vi "WS102x FPGA Multi DUT Reliability Ver1.1.vi"() -> ()   [LabVIEW 2017]
uses:
  Type Def/Test Sequences.ctl
  WS_VCAP Driver 039/Source/WSVCAP Shell/Type Defs/WSVCAP SHL FPGA Enum.ctl
  <vilib>/userdefined/High Color/nirio_resource_hc.ctl
  WS_VCAP Driver 039/Source/WSVCAP Shell/Type Defs/WSVCAP SHL I2C DUT Mask Mode Enum.ctl
  <vilib>/Utility/error.llb/whitespace.ctl
  <vilib>/Utility/file.llb/Read Delimited Spreadsheet (DBL).vi
panel:
  in  "Main":T1(tab)
  in  "Clock Rate Meas(Hz)":dbl=1000000.0 format="%.1p Hz"
  in  "CAPDAC Value":u8=128 format="0x%02x"
  in  "DUT Mask Mode (All)":T2=enum."All"
  in  "SN Brd B":string[](array[string])=["1", "2", "3", "4", "5", "6", "7", "8", "9", "10", "11", "12", "13", "14", "15", "16", "17", "18", "19", "20", "21", "22", "23", "24", "25", "26", "27", "28", "29", "30", "31", "32"]
  in  "SN Brd A":string[](array[string])=["1", "2", "3", "4", "5", "6", "7", "8", "9", "10", "11", "12", "13", "14", "15", "16", "17", "18", "19", "20", "21", "22", "23", "24", "25", "26", "27", "28", "29", "30", "31", "32"]
  in  "Info Brd B":T3={"Lot #"="1K3CB", "Wafer #"="19", "Board"="B", "Comment"="CYC 45C 44V", "File Name"="CYC_1K3CB_19WO_25C_44V_25DC_Brd2B_190124_1", "Data File Path Control"=path "C:/WS102x 32 DUT Data"}
  in  "Info Brd A":T3={"Lot #"="1K3CB", "Wafer #"="19", "Board"="A", "Comment"="CYC 45C 44V", "File Name"="CYC_1K3CB_19_WO_25C_44V_25DC_Brd2A_190124_1", "Data File Path Control"=path "C:/WS102x 32 DUT Data"}
  in  "Test Program":string="WS102x FPGA Multi DUT Reliability Ver1.1"
  in  "Calibration AD":bool
  in  "Initialize ADI":bool
  in  "Data Brd B?":bool=TRUE
  in  "Data Brd A?":bool=TRUE
  in  "Setup Test":T4(tab)
  in  "Manual Command":string
  in  "Verify Beams":bool
  in  "Manual Setting":i32(ring) items=["CP OFF", "CP ON", "OTP OFF", "CP 24V", "CP 26V", "CP 28V", "CP 30V", "CP 31V", "CP 32V", "CP 33V", "CP 34V", "CP 35V", "CP 36V", "CP 37V", "CP 38V", "CP 39V", "CP 40V", "CP 41V", "CP 42V", "CP 43V", "CP 44V", "CP 45V", "CP 46V", "CP 47V", "CP 48V", "CP 49V", "CP 50V", "CP 51V", "CP 52V", "CP 53V", "CP 54V", "CP 56V", "CP 58V", "CP 60V", "CP 62V"]
  in  "CP Measurement":i32(ring)=20 items=["CP OFF", "CP ON", "OTP OFF", "CP 24V", "CP 26V", "CP 28V", "CP 30V", "CP 31V", "CP 32V", "CP 33V", "CP 34V", "CP 35V", "CP 36V", "CP 37V", "CP 38V", "CP 39V", "CP 40V", "CP 41V", "CP 42V", "CP 43V", "CP 44V", "CP 45V", "CP 46V", "CP 47V", "CP 48V", "CP 49V", "CP 50V", "CP 51V", "CP 52V", "CP 53V", "CP 54V", "CP 56V", "CP 58V", "CP 60V", "CP 62V"]
  in  "Select CP VPI":i32(ring)=16 items=["CP OFF", "CP ON", "OTP OFF", "CP 24V", "CP 26V", "CP 28V", "CP 30V", "CP 31V", "CP 32V", "CP 33V", "CP 34V", "CP 35V", "CP 36V", "CP 37V", "CP 38V", "CP 39V", "CP 40V", "CP 41V", "CP 42V", "CP 43V", "CP 44V", "CP 45V", "CP 46V", "CP 47V", "CP 48V", "CP 49V", "CP 50V", "CP 51V", "CP 52V", "CP 53V", "CP 54V", "CP 56V", "CP 58V", "CP 60V", "CP 62V"]
  in  "Select CP Stress":i32(ring)=20 items=["CP OFF", "CP ON", "OTP OFF", "CP 24V", "CP 26V", "CP 28V", "CP 30V", "CP 31V", "CP 32V", "CP 33V", "CP 34V", "CP 35V", "CP 36V", "CP 37V", "CP 38V", "CP 39V", "CP 40V", "CP 41V", "CP 42V", "CP 43V", "CP 44V", "CP 45V", "CP 46V", "CP 47V", "CP 48V", "CP 49V", "CP 50V", "CP 51V", "CP 52V", "CP 53V", "CP 54V", "CP 56V", "CP 58V", "CP 60V", "CP 62V"]
  in  "VDD":dbl=3.3 format="%.2g"
  in  "CP Setting":bool
  in  "Cycle DC %":string="25"
  in  "Set Delay Speed":dbl[](array[numeric])=[1.7e-05, 4.9e-05] min=0.0 max=0.5 format="%#.0p s"
  in  "Cycling Bit":string[](array[string])=["0701027F7F", "0701020000"]
  out "Stress DC(%)":string
  in  "HD Beams":string="ALL Beams"
  in  "HD Cmd":string="0701027F7F"
  in  "Test Condition Setting":T5={"Freq (KHz)"="12", "ACV (V)"="0", "AC Freq (Hz)"="0", "Temp (C)"="25", "DCV (V)"=0.0, "CYC RP (x1000)"=10000, "HD RP (Min)"=60, "RPM Delay (s)"=60, "Select VCmin"=2} {"Select VCmin" items=["FBs", "TBs", "ALL"]}
  out "Test Run Selected":T6
  in  "Test Run Setting":T7={"OTP ?  "=FALSE, "STRESS ?  "=TRUE, "VPI ?  "=TRUE, "OPEN STATE VCMIN ?  "=TRUE, "CLOSE STATE VCMIN ?  "=TRUE, "RPM (Verify Socket) ?  "=FALSE, "HS CHK?"=TRUE}
  out "Data Board B":string[][](array[string])
  in  "Stop":bool
  out "Current Time":string
  out "Current Date":string
  in  "Start Date":string
  in  "Start Time":string
  in  "Select Measurement":i32(ring) items=["Temperature", "Humidity", "TH1", "TH2"]
  out "Temp (C)":string
  out "RH(%)":string
  out "Test Sequences":T8
  out "Error Out":errorcluster
  in  "Error In":errorcluster
  in  "Start":bool
  out "Data Board A":string[][](array[string])
  out "AD7747 Value Brd B":string[][](table)=[["Device", "Status", "Cap (pF)", "SN"], ["DUT 01", "", "", "01"], ["DUT 02", "", "", "02"], ["DUT 03", "", "", "03"], ["DUT 04", "", "", "04"], ["DUT 05", "", "", "05"], ["DUT 06", "", "", "06"], ["DUT 07", "", "", "07"], ["DUT 08", "", "", "08"], ["DUT 09", "", "", "09"], ["DUT 10", "", "", "10"], ["DUT 11", "", "", "11"], ["DUT 12", "", "", "12"], ["DUT 13", "", "", "13"], ["DUT 14", "", "", "14"], ["DUT 15", "", "", "15"], ["DUT 16", "", "", "16"], ["DUT 17", "", "", "17"], ["DUT 18", "", "", "18"], ["DUT 19", "", "", "19"], ["DUT 20", "", "", "20"], ["DUT 21", "", "", "21"], ["DUT 22", "", "", "22"], ["DUT 23", "", "", "23"], ["DUT 24", "", "", "24"], ["DUT 25", "", "", "25"], ["DUT 26", "", "", "26"], ["DUT 27", "", "", "27"], ["DUT 28", "", "", "28"], ["DUT 29", "", "", "29"], ["DUT 30", "", "", "30"], ["DUT 31", "", "", "31"], ["DUT 32", "", "", "32"]]
  out "AD7747 Value Brd A":string[][](table)=[["Device", "Status", "Cap (pF)", "SN"], ["DUT 01", "", "", "01"], ["DUT 02", "", "", "02"], ["DUT 03", "", "", "03"], ["DUT 04", "", "", "04"], ["DUT 05", "", "", "05"], ["DUT 06", "", "", "06"], ["DUT 07", "", "", "07"], ["DUT 08", "", "", "08"], ["DUT 09", "", "", "09"], ["DUT 10", "", "", "10"], ["DUT 11", "", "", "11"], ["DUT 12", "", "", "12"], ["DUT 13", "", "", "13"], ["DUT 14", "", "", "14"], ["DUT 15", "", "", "15"], ["DUT 16", "", "", "16"], ["DUT 17", "", "", "17"], ["DUT 18", "", "", "18"], ["DUT 19", "", "", "19"], ["DUT 20", "", "", "20"], ["DUT 21", "", "", "21"], ["DUT 22", "", "", "22"], ["DUT 23", "", "", "23"], ["DUT 24", "", "", "24"], ["DUT 25", "", "", "25"], ["DUT 26", "", "", "26"], ["DUT 27", "", "", "27"], ["DUT 28", "", "", "28"], ["DUT 29", "", "", "29"], ["DUT 30", "", "", "30"], ["DUT 31", "", "", "31"], ["DUT 32", "", "", "32"]]
  in  "Instruments":T10={"KE2400"="GPIB0::3::INSTR", "KE2000"="GPIB0::9::INSTR", "Agilent P/S"="GPIB0::5::INSTR", "Temperature Sensor"="", "FPGA"=enum."RIO0"}
  out "Activity Log":string
  out "FPGA Resource":T11
  out "Online":bool
  out "Simulate FPGA":bool
  in  "RFFE Slave Address":u8=7 caption="Slave Address" format="0x%02x"
  in  "Clock Rate Cycle(Hz)":dbl=5000000.0 format="%.1p Hz"
  out "Error Status":string
  out "IDD Measurement(uA)":string[](array[string])
  out "Cycle Count":u64=2 min=1 max=4 step=1
  out "Status":string
  out "Last Run Time":string
  out "Last Run Date":string
  out "T0_Brd B Delta C%":string[](array[string])
  out "T0_Brd A Delta C%":string[](array[string])
  in  "Abort Stress":bool
  out "TTF Completed":u64
  in  "Set TTF":u64=50000000000
  out "Brd B_VPI Cap (fF)":string[][](table)
  out "Brd B_Beam Cap (fF)":string[][](table)
  out "Brd A_VPI Cap (fF)":string[][](table)
  out "Brd A_Beam Cap (fF)":string[][](table)
  out "Verify CP Stress":string[](array[string])
  out "Brd B Pass/Fail?":bool[](array[boolean])
  out "Brd A Pass/Fail?":bool[](array[boolean])
  out "Verify DC Speed":dbl[](array[numeric]) format="%#.0p s"
  out "Verify Bits to Cycle":string[](array[string])
  out "Brd A Delta C%":string[](array[string])
  out "Brd B Delta C%":string[](array[string])
  out "Brd B_OS_V3 (fF)":string[][](table)
  out "Brd B_OS_V2 (fF)":string[][](table)
  out "Brd B_OS_V1 (fF)":string[][](table)
  in  "OS_Voltage(V)":dbl[](array[numeric])=[-10.0, 0.0, 10.0]
  out "Brd A_OS_V3 (fF)":string[][](table)
  out "Brd A_OS_V2 (fF)":string[][](table)
  out "Brd A_OS_V1 (fF)":string[][](table)
  out "VPI Brd B Delta C%":string[](array[string])
  out "VPI Brd A Delta C%":string[](array[string])
  out "Cmin BrdB":string[](array[string])
  out "Cmin BrdA":string[](array[string])
  out "RB for HD Stress":string[][](array[string])
  out "Brd B_CS_V3 (fF)":string[][](table)
  out "Brd B_CS_V2 (fF)":string[][](table)
  out "Brd B_CS_V1 (fF)":string[][](table)
  out "Brd A_CS_V3 (fF)":string[][](table)
  out "Brd A_CS_V2 (fF)":string[][](table)
  out "Brd A_CS_V1 (fF)":string[][](table)
  in  "CS_Voltage(V)":dbl[](array[numeric])=[-3.0, 0.0, 3.0]
  out "CMin BrdA (fF)":dbl[](array[numeric])
  out "CMin BrdB (fF)":dbl[](array[numeric])
  out "Brd B_CS VCmin":string[][](table)
  out "Brd A_CS VCmin":string[][](table)
  out "Brd B_CS VCmin_T0":string[][](table)
  out "Brd A_CS VCmin_T0":string[][](table)
  in  "Col CMin":i32=23
  out "Board B":dbl[][](graph)
  out "Board A":dbl[][](graph)
  in  "Plot":T12(ring)
  # "Company: WiSpry Inc Powered by AAC Technologies\n20 Fairbanks Suite 198, Irvine CA 92618\n\nCreated Date:  02-22-2019\nTP:  WS1021 32 DUT Board, Reliability Ver1.1\nFPGA Modular:  WS_VCAP_Driver 039"
  # "WS1021 FPGA 32 DUT Reliability Ver1.0\n\nVer1.0:  Original Version for HD only (1-24-2019)\nVer1.1:  Updated from Version 1.0 for both HD or Cycliing runs (2-22-2019)"
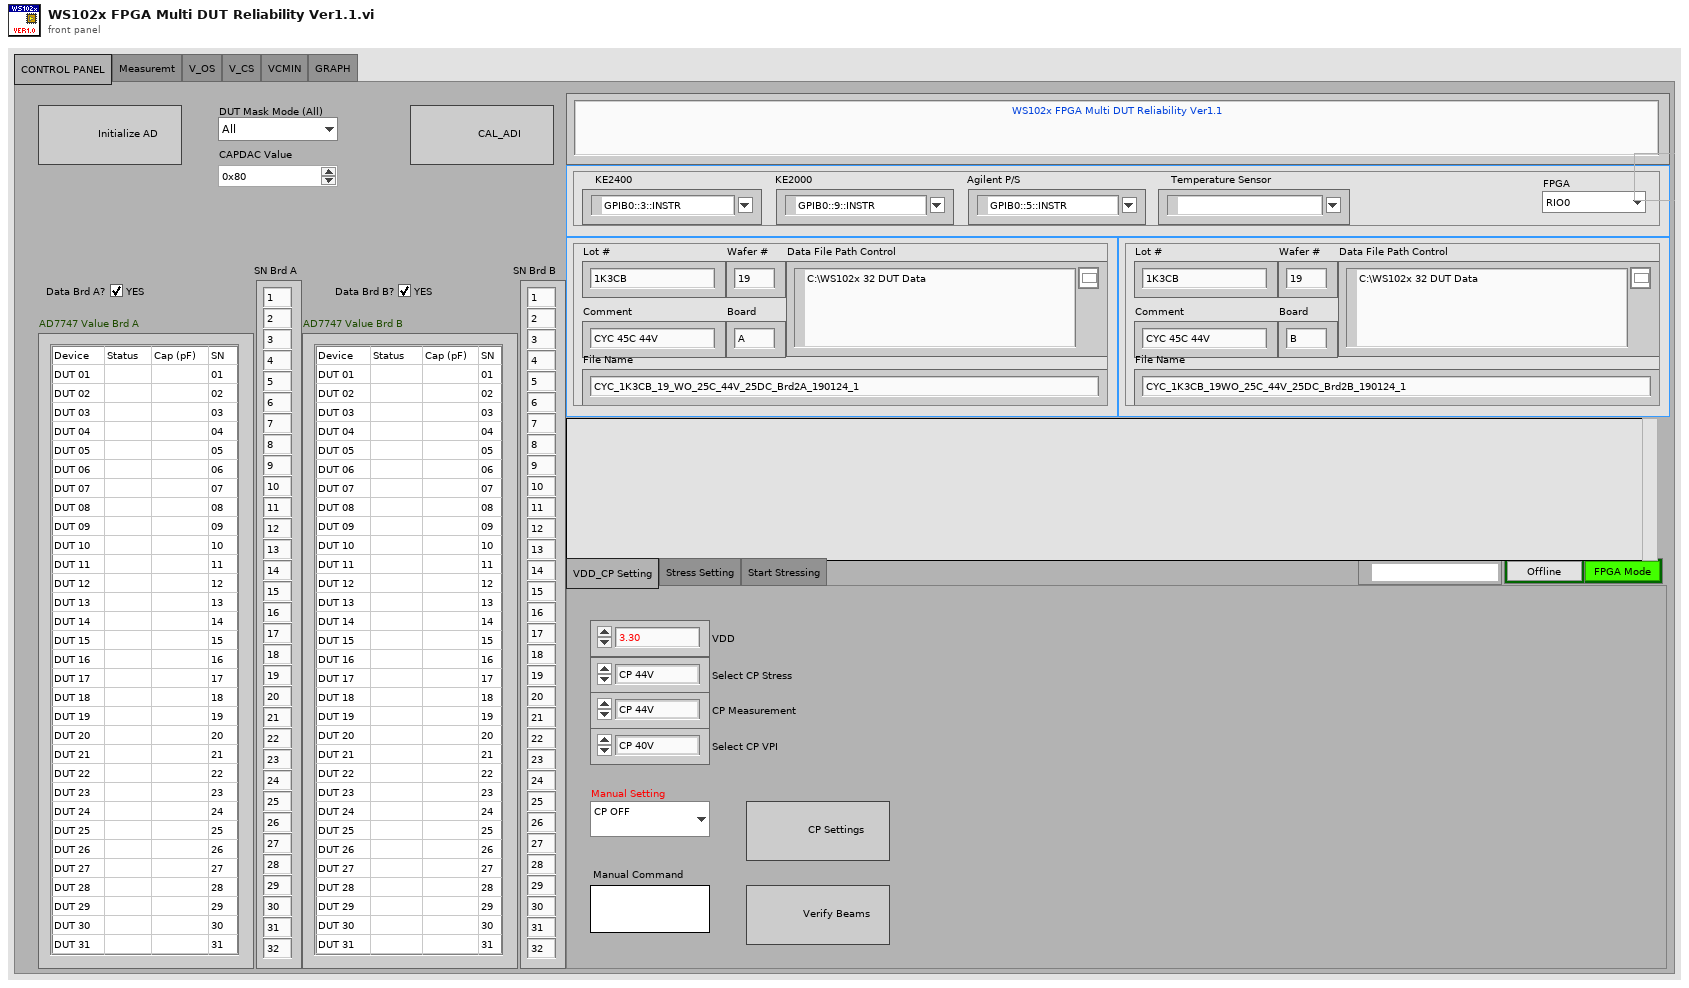
[diagram p1: front panel]
types:
  T1 = enum32{"CONTROL PANEL", "Measuremt", "V_OS", "V_CS", "VCMIN", "GRAPH"}
  T2 = typedef "WSVCAP SHL I2C DUT Mask Mode Enum.ctl" = enum16{"Custom", "All"}
  T3 = cluster{"Lot #":string, "Wafer #":string, "Board":string, "Comment":string, "File Name":string, "Data File Path Control":path}
  T4 = enum32{"VDD_CP Setting", "Stress Setting", "Start Stressing"}
  T5 = cluster{"Freq (KHz)":string, "ACV (V)":string, "AC Freq (Hz)":string, "Temp (C)":string, "DCV (V)":dbl, "CYC RP (x1000)":u64, "HD RP (Min)":u64, "RPM Delay (s)":u64, "Select VCmin":u16}
  T6 = cluster{"OTP":bool, "CYC/HD":bool, "VPI":bool, "OSV":bool, "CSV":bool, "RPM":bool, "HS CHK":bool}
  T7 = cluster{"OTP ?  ":bool, "STRESS ?  ":bool, "VPI ?  ":bool, "OPEN STATE VCMIN ?  ":bool, "CLOSE STATE VCMIN ?  ":bool, "RPM (Verify Socket) ?  ":bool, "HS CHK?":bool}
  T8 = typedef "Test Sequences.ctl" = enum16{"VDD", "CP Setting", "HS CHK", "Stress", "I_Measure", "Cap_Measure", "VPI", "Open State VCmin", "Close State VCmiin", "Save Data", "Exit"}
  T9 = typedef "WSVCAP SHL FPGA Enum.ctl" = enum16{"RIO0", "RIO1"}
  T10 = cluster{"KE2400":refnum<visa-resource-name>, "KE2000":refnum<visa-resource-name>, "Agilent P/S":refnum<visa-resource-name>, "Temperature Sensor":refnum<visa-resource-name>, "FPGA":T9}
  T11 = typedef "nirio_resource_hc.ctl" = tag
  T12 = enum16{"ALL DUTs", "DUT 01", "DUT 02", "DUT 03", "DUT 04", "DUT 05", "DUT 06", "DUT 07", "DUT 08", "DUT 09", "DUT 10", "DUT 11", "DUT 12", "DUT 13", "DUT 14", "DUT 15", "DUT 16", "DUT 17", "DUT 18", "DUT 19", "DUT 20", "DUT 21", "DUT 22", "DUT 23", "DUT 24", "DUT 25", "DUT 26", "DUT 27", "DUT 28", "DUT 29", "DUT 30", "DUT 31", "DUT 32"}
  T13 = enum16{"Idle...", "Voltage 1", "Voltage 2", "Voltage 3"}
  T14 = typedef "WSVCAP SHL Core System Cluster.ctl" = cluster{"Settings":T15, "FPGA Resource":tag, "Online":bool, "I2C Wait Ticks":u32, "SPI Wait Ticks":u32, "RFFE Wait Ticks":u32, "FPGA VI Reference (FPGA Mode)":T16, "FPGA VI Reference (Sim Mode)":refnum<vi>}
  T15 = typedef "WSVCAP SHL I2C Settings Cluster.ctl" = cluster{"I2C Slave Address":u8, "I2C Clock Rate (Hz)":dbl, "SPI Clock Rate (Hz)":dbl, "RFFE Slave Address":u8, "RFFE Clock Rate (Hz)":dbl, "Simulate FPGA":bool, "C1 Cap DAC Default":u8, "C2 Cap DAC Default":u8, "C3 Cap DAC Default":u8, "C4 Cap DAC Default":u8}
  T16 = typedef "WSVCAP SHL FPGA Ref.ctl" = refnum<k20>
  T17 = enum16{"Idle...", "Voltage 1", "Voltage 2", "Voltage 3"}[]
  T18 = typedef "whitespace.ctl" = u16
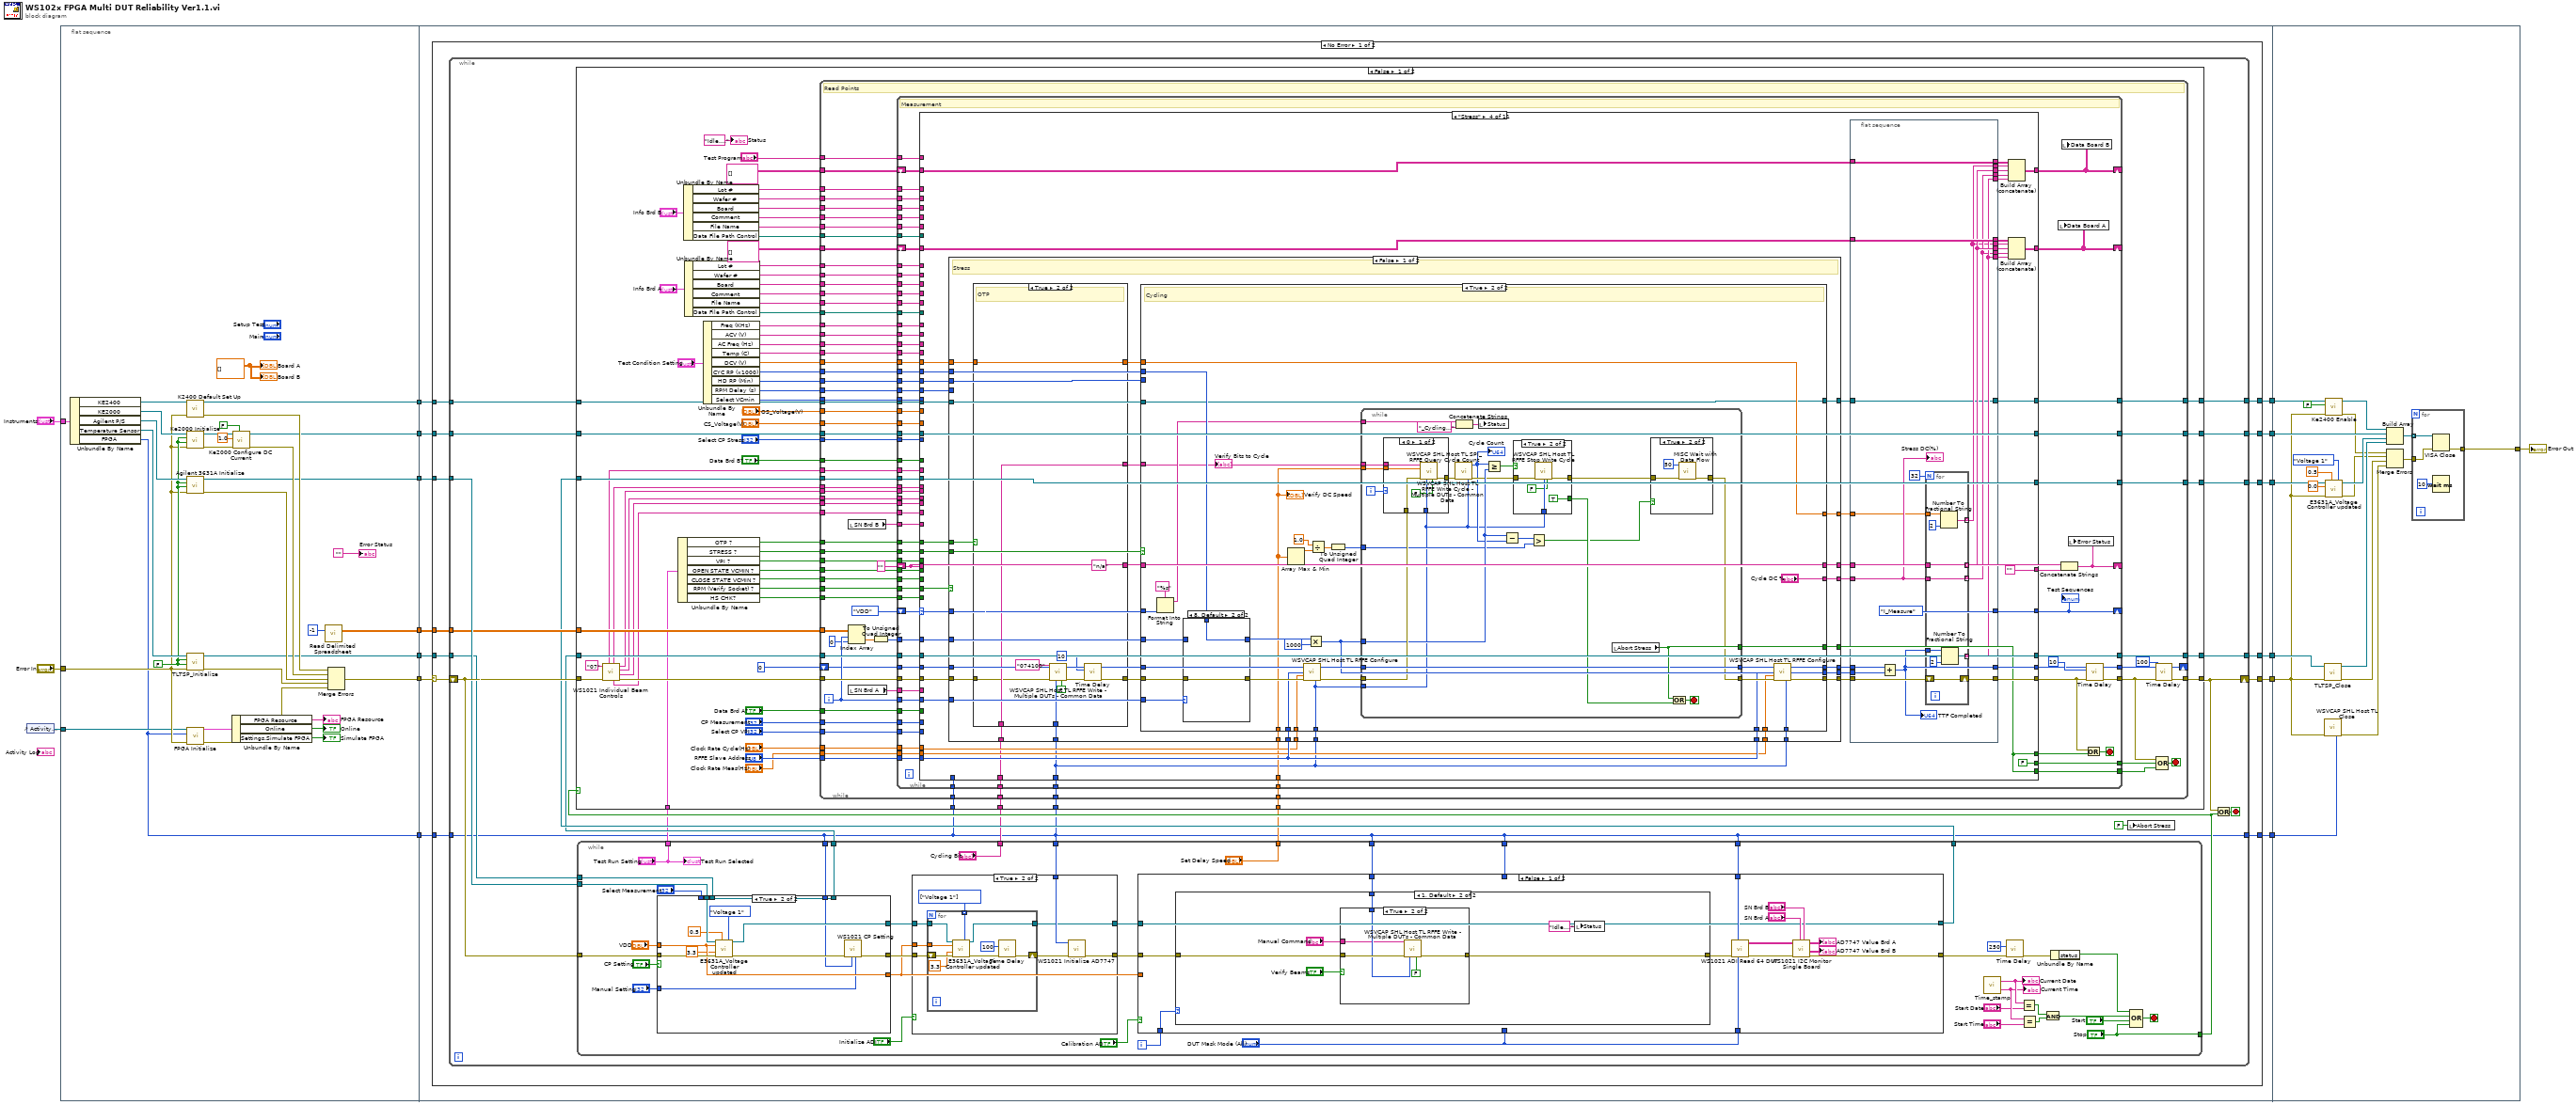
[diagram p0: block diagram]
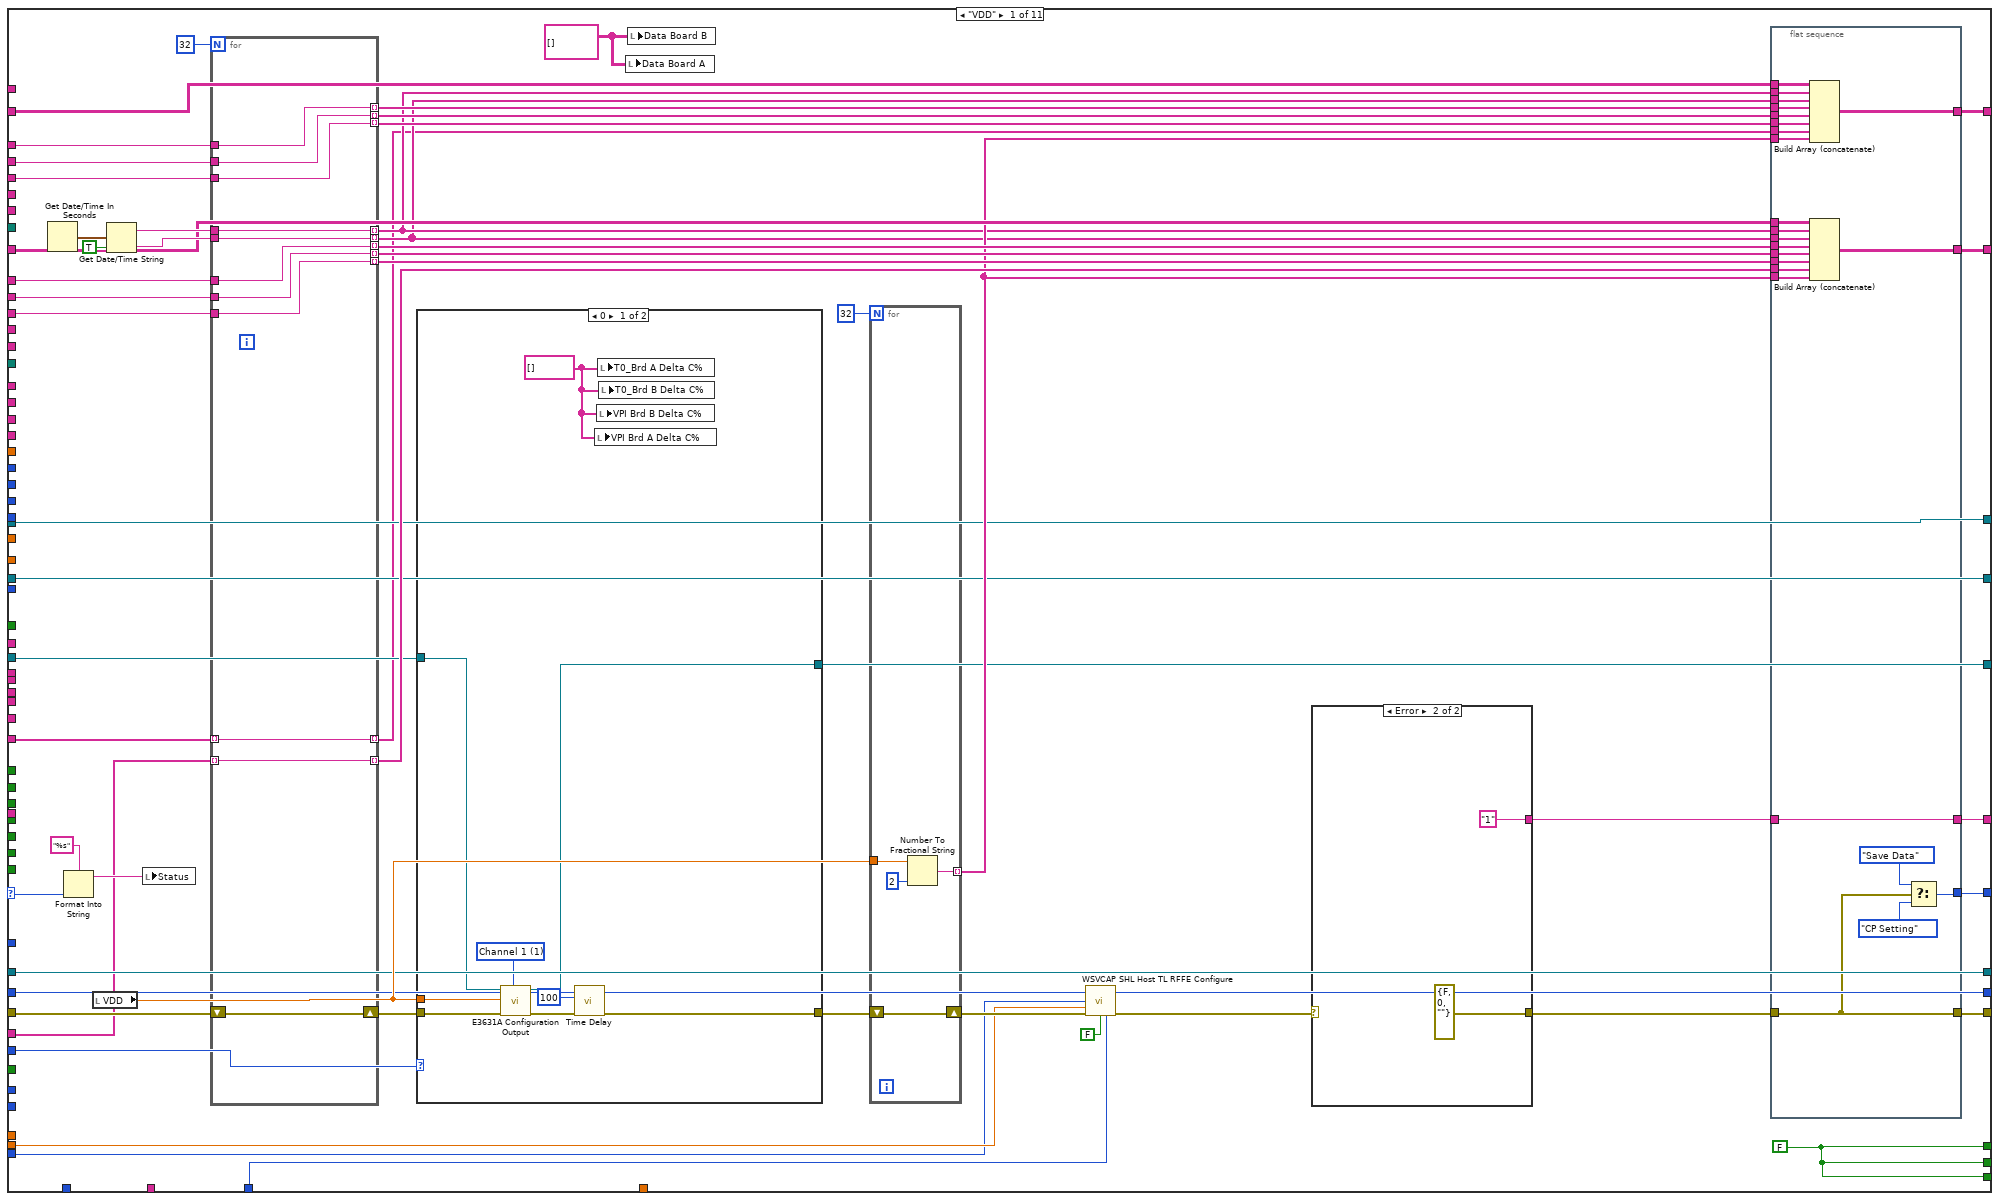
[diagram p2: hidden frame]
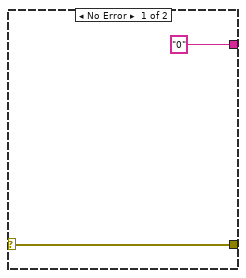
[diagram p3: hidden frame]
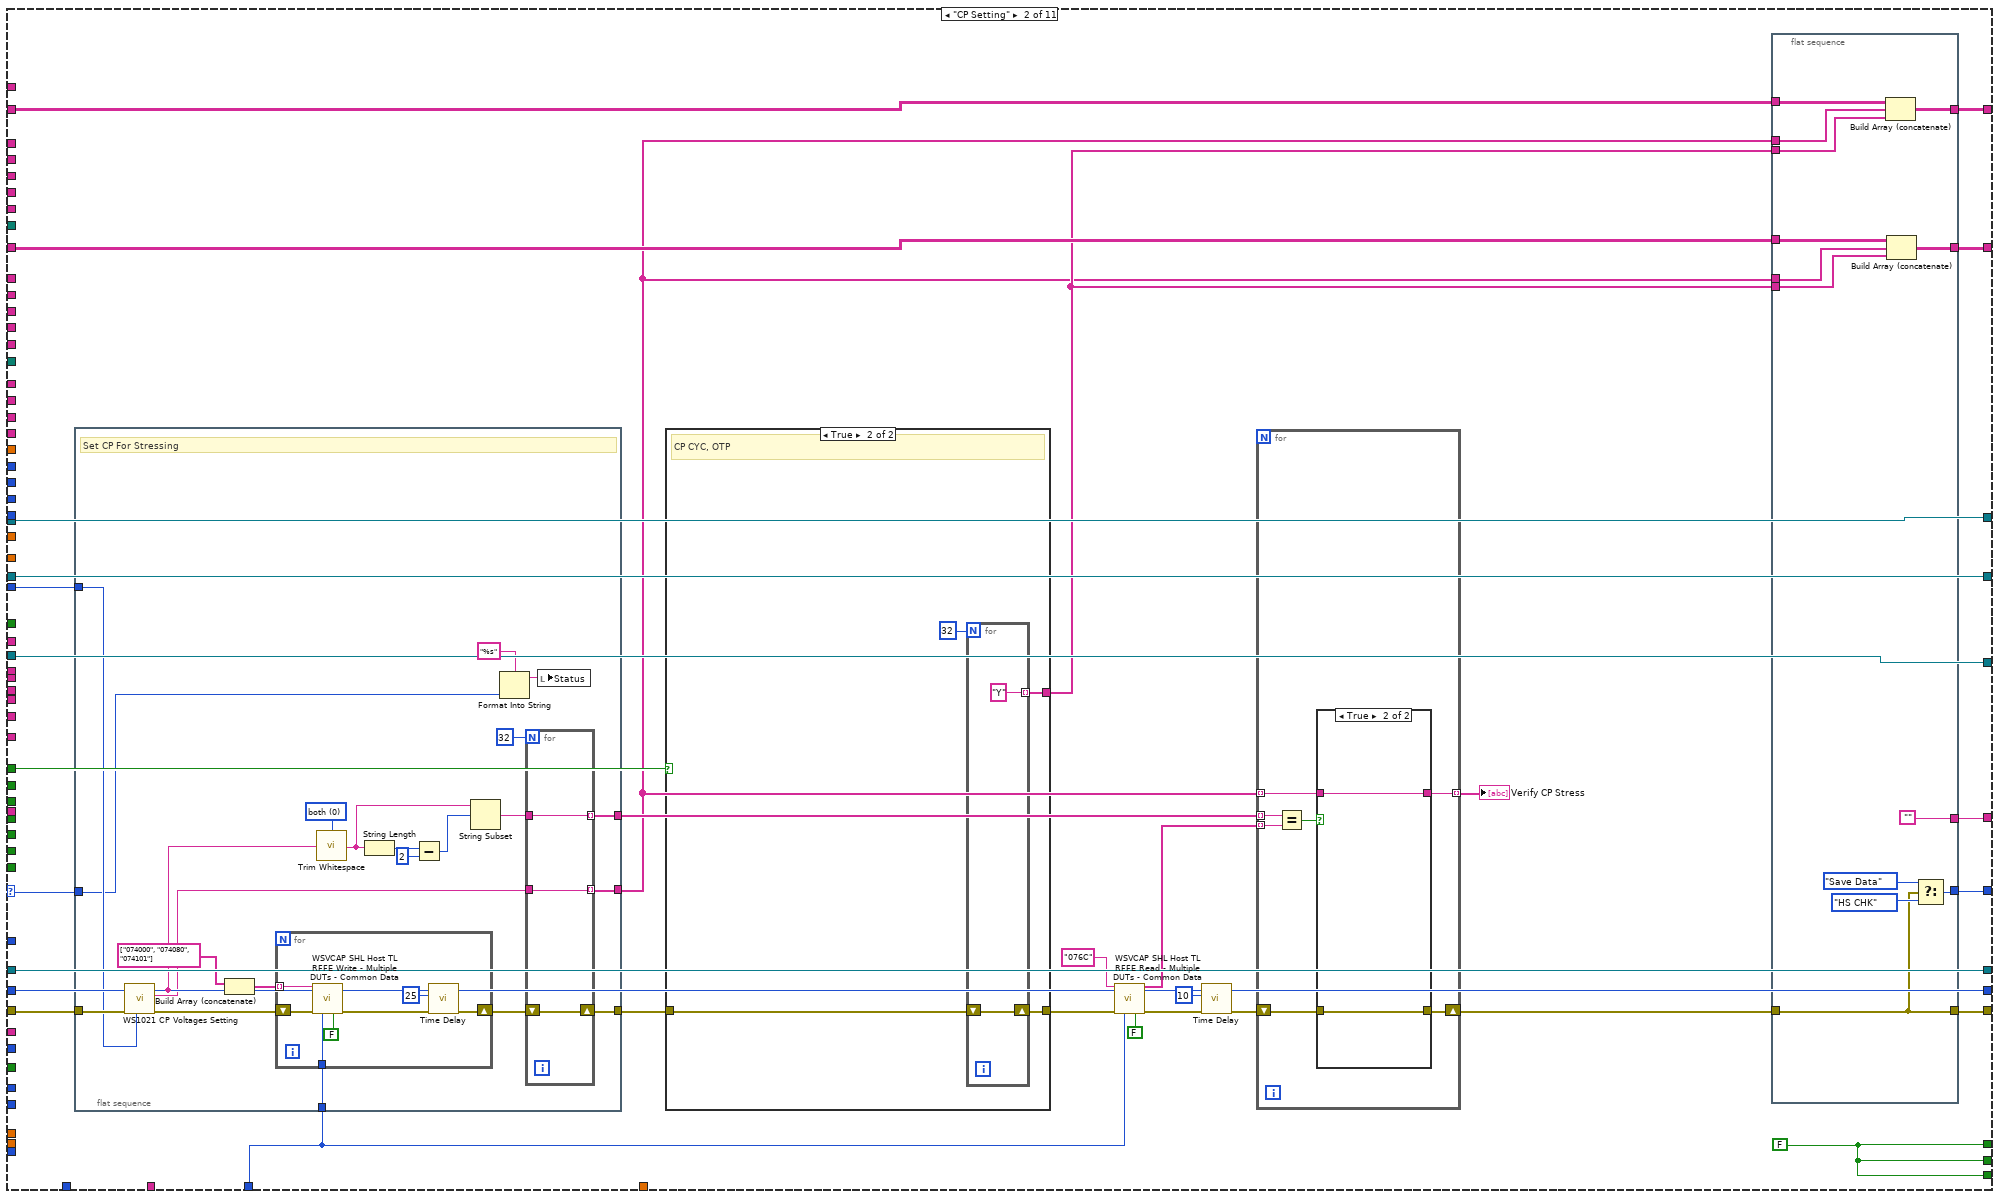
[diagram p5: hidden frame]
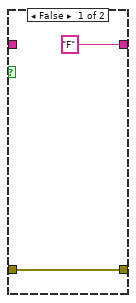
[diagram p6: hidden frame]
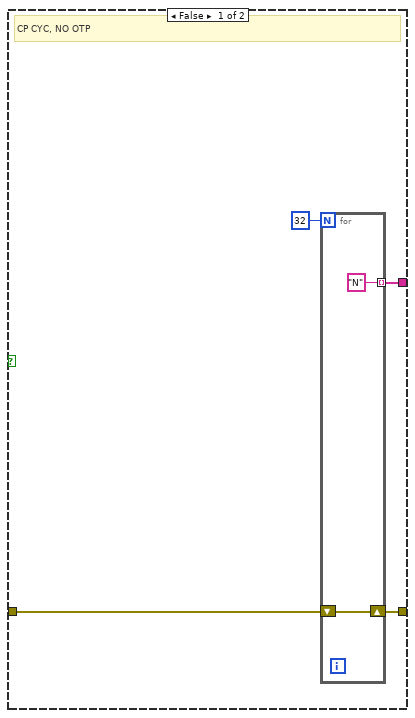
[diagram p7: hidden frame]
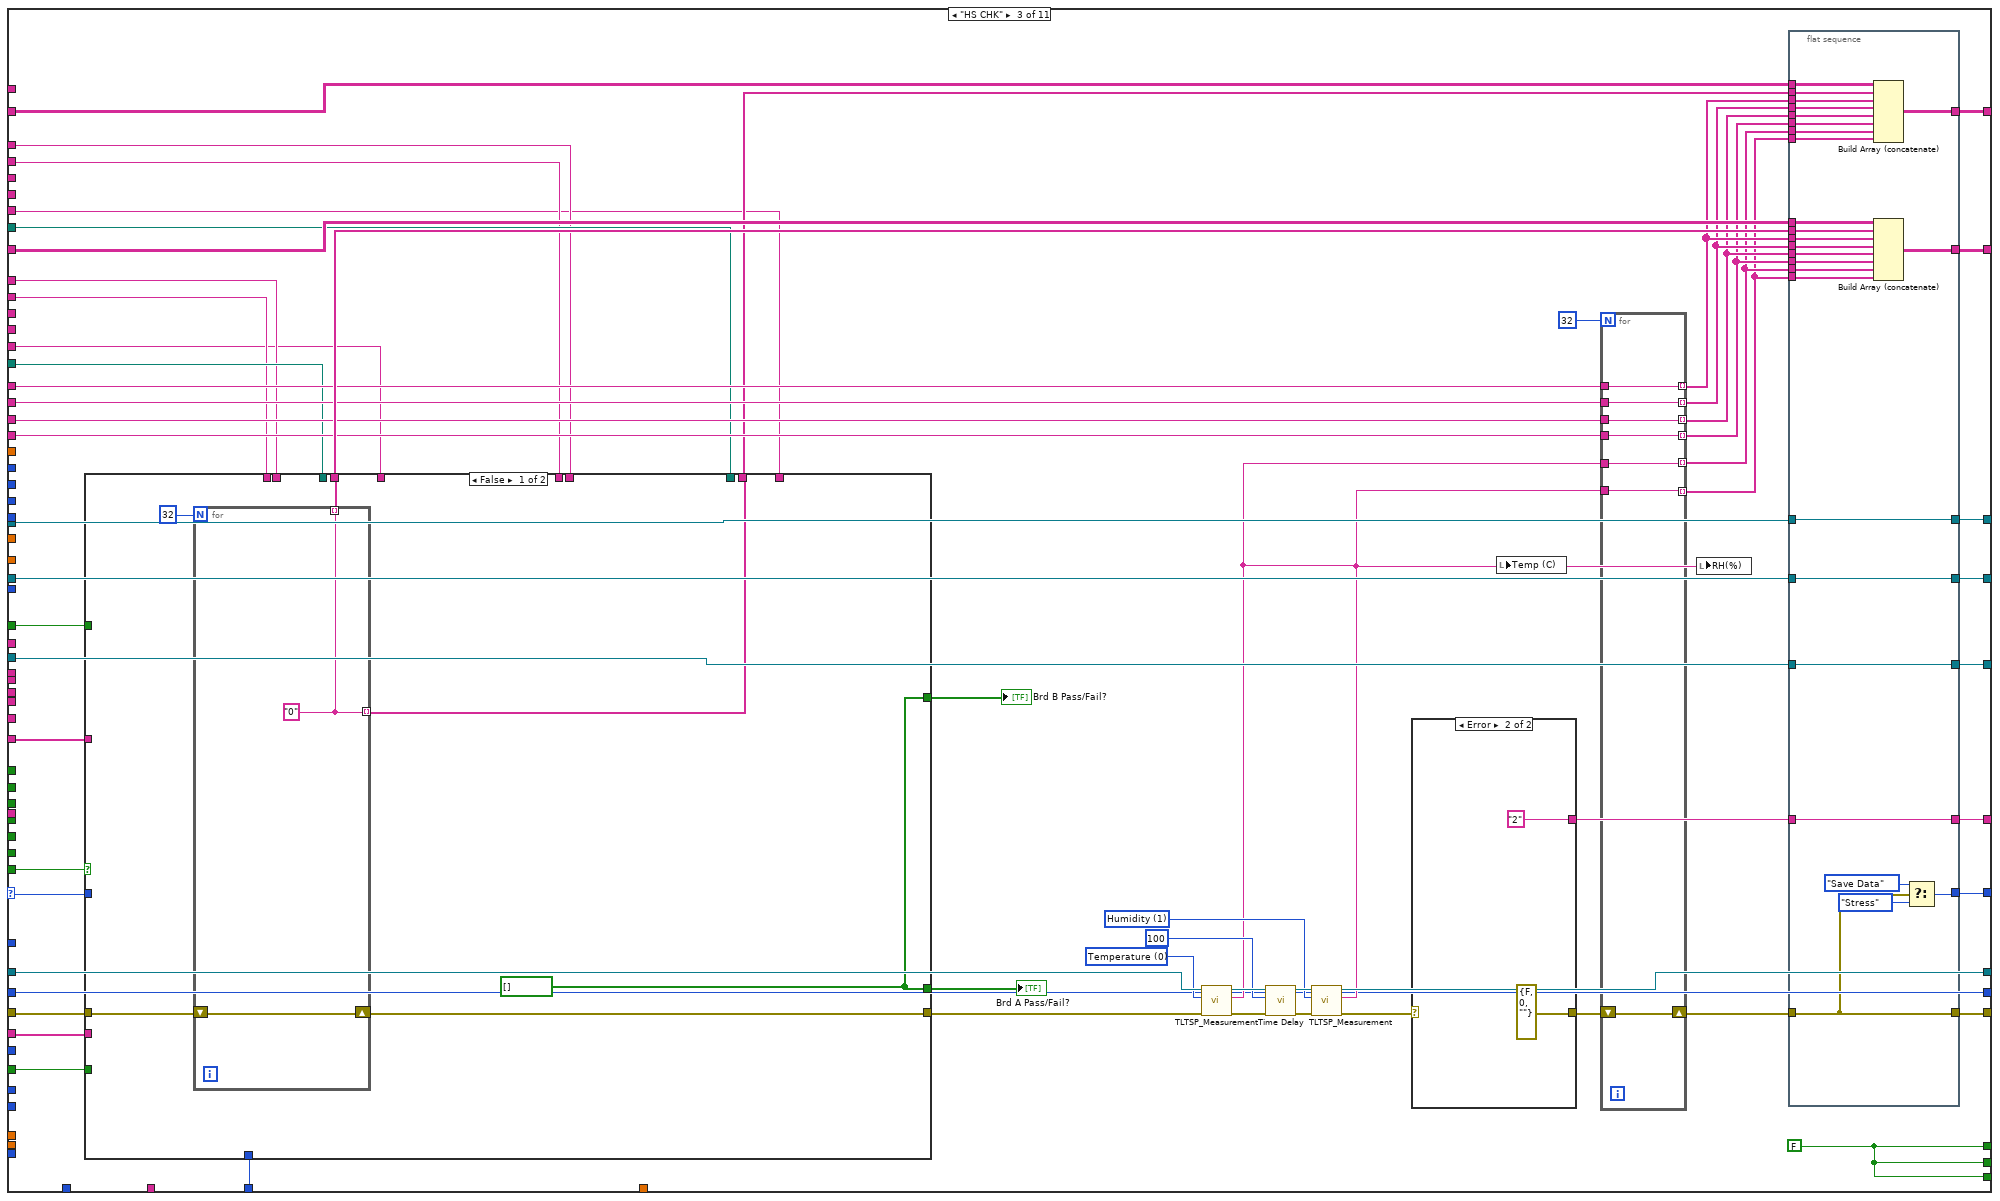
[diagram p8: hidden frame]
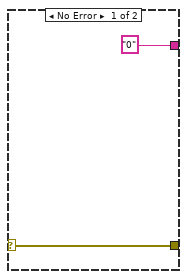
[diagram p9: hidden frame]
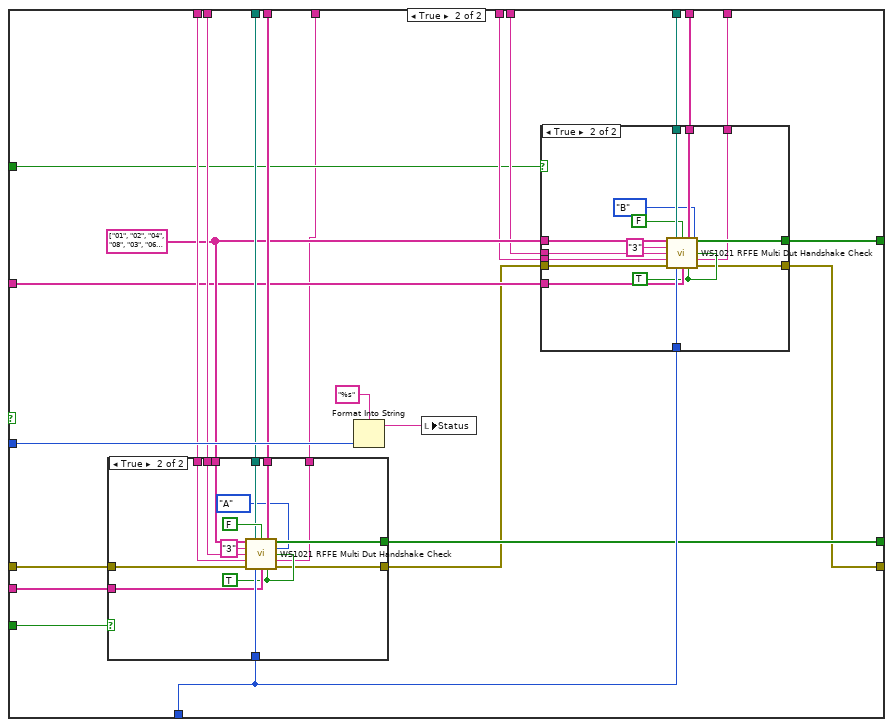
[diagram p10: hidden frame]
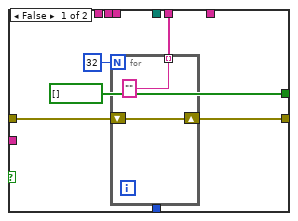
[diagram p11: hidden frame]
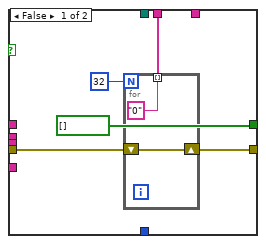
[diagram p12: hidden frame]
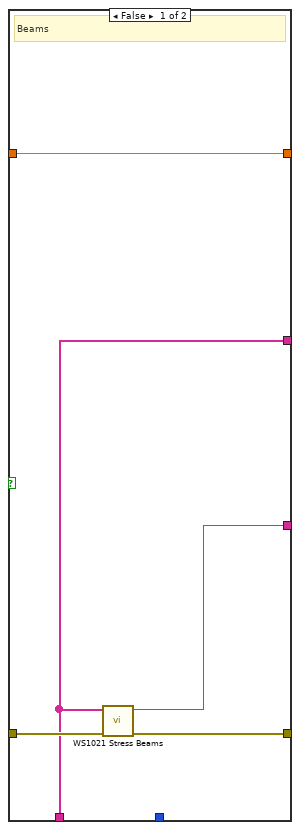
[diagram p13: hidden frame]
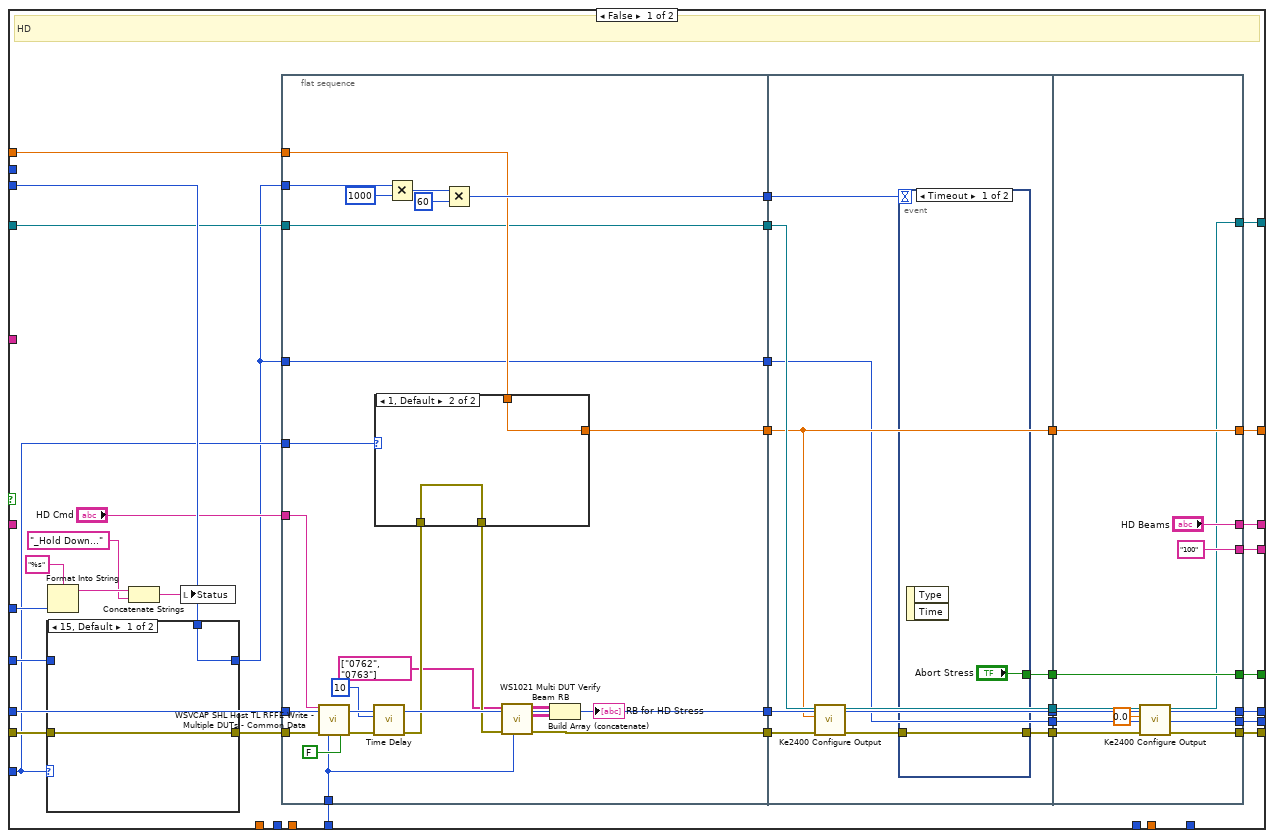
[diagram p14: hidden frame]
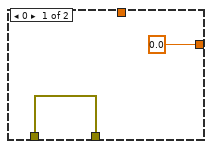
[diagram p16: hidden frame]
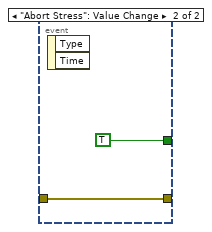
[diagram p17: hidden frame]
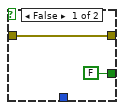
[diagram p20: hidden frame]
diagram:
  n1 = control-ref of="Activity Log"() -> (w3:refnum<vi>)
  n2 = flat-sequence {
    tunnel: [w35] -> w17
    tunnel: "Instruments" -> [w48]
    tunnel: "Error In" -> [w26]
    tunnel: [w32] -> w12
    tunnel: [w31] -> w11
    tunnel: [w30] -> w10
    tunnel: [w29] -> w9
    tunnel: [w27] -> w4
    tunnel: w3 -> [w24]
    tunnel: [w19] -> w2
    tunnel: w17 -> [w61]
    tunnel: [w60] -> w16
    tunnel: w12 -> [w59]
    tunnel: w11 -> [w58]
    tunnel: w10 -> [w57]
    tunnel: w9 -> [w56]
    tunnel: [w55] -> w8
    tunnel: [w54] -> w7
    tunnel: [w53] -> w6
    tunnel: [w52] -> w5
    tunnel: w4 -> [w51]
    tunnel: w2 -> [w50]
    tunnel: [w49] -> w1
    tunnel: w16 -> [w2137]
    tunnel: [w2138] -> w15
    tunnel: w8 -> [w2153]
    tunnel: w7 -> [w2149]
    tunnel: w6 -> [w2146]
    tunnel: w5 -> [w2154]
    tunnel: w1 -> [w2136]
    frame #0 {
      w42 = FALSE ("Reset")
      w47 = dbl[][] [] ("Board 1")
      n3 = Unbundle By Name(w48) -> ("KE2400"=w46:refnum<visa-resource-name>, "KE2000"=w45:refnum<visa-resource-name>, "Agilent P/S"=w44:refnum<visa-resource-name>, "Temperature Sensor"=w43:refnum<visa-resource-name>, "FPGA"=w19:T9)
      n4 = call "K2400 Default Set Up.vi"("Error In"=w26, "Ke2400 In"=w46) -> ("Error Out"=w39:errorcluster, "Ke2400 Out"=w32:refnum<visa-resource-name>)  [unwired: 8 in]
      n5 = call "Ke2000 Initialize.vi"("error in (no error)"=w26, "Default Setting"=w42, "Reset"=w42, "VISA resource name"=w45) -> ("error out"=w40:errorcluster, "VISA resource name out"=w41:refnum<visa-resource-name>)  [unwired: 6 in]
      n6 = call "Agilent 3631A Initialize.vi"("error in (no error)"=w26, "Default"=w42, "Reset"=w42, "VISA resource name"=w44) -> ("error out"=w37:errorcluster, "VISA resource name out"=w30:refnum<visa-resource-name>)  [unwired: 6 in]
      n7 = call "TLTSP_Initialize.vi"("error in (no error)"=w26, "Query ID?"=w42, "Reset"=w42, "VISA In"=w43) -> ("error out"=w36:errorcluster, "VISA Out"=w29:refnum<visa-resource-name>)  [unwired: 5 in, 1 out]
      n8 = call "FPGA Initialize.vi"("Error In"=w26, "FPGA"=w19, "Active Log"=w24) -> ("Error Out"=w25:errorcluster, "System Out"=w23:T14)  [unwired: 7 in]
      n9 = Unbundle By Name(w23) -> ("FPGA Resource"=→"FPGA Resource":tag, "Online"=→"Online":bool, "Settings.Simulate FPGA"=→"Simulate FPGA":bool)
      n10 = call "Ke2000 Configure DC Current.vi"("Auto Range? (T: Auto)"=FALSE, "error in"=w40, "Custom Range (0 A)"=1.0, "VISA resource name"=w41) -> ("error out"=w38:errorcluster, "VISA resource name out"=w31:refnum<visa-resource-name>)  [unwired: 6 in]
      n11 = call-poly <vilib>:"Read Delimited Spreadsheet.vi"("number of rows (all:-1)"=-1) -> ("all rows"=w27:dbl[][])  [unwired: 9 in, 5 out]
      n12 = Merge Errors(w39, w38, w37, w36, w25) -> (w35:errorcluster)
      "Board B" <- w47
      "Board A" <- w47
      "Error Status" <- ""
    }
    frame #1 {
      n13 = case shown="No Error" w61 {
        selector: w61 -> [w73 w2131]
        tunnel: [w74 w2130] -> w60
        tunnel: w59 -> [w72 w2129]
        tunnel: w58 -> [w71 w2128]
        tunnel: w57 -> [w70 w2127]
        tunnel: w56 -> [w69 w2126]
        tunnel: [w68 w2127] -> w55
        tunnel: [w67 w2129] -> w54
        tunnel: [w66 w2128] -> w53
        tunnel: [w65 w2126] -> w52
        tunnel: w51 -> [w64 _]
        tunnel: w50 -> [w63 w2125]
        tunnel: [w62 w2125] -> w49
        frame No Error {
          n14 = while {
            shift-right: [w92] -> w74
            shift-left: w73 -> [w94]
            tunnel: w72 -> [w90]
            tunnel: w71 -> [w89]
            tunnel: w70 -> [w88]
            tunnel: w69 -> [w82]
            tunnel: [w87] -> w68
            tunnel: [w86] -> w67
            tunnel: [w85] -> w66
            tunnel: [w84] -> w65
            tunnel: w64 -> [w83]
            tunnel: w63 -> [w75]
            tunnel: [w75] -> w62
            stop <- w93 stop-if-true
            n15 = while {
              tunnel: w94 -> [w2010]
              tunnel: ["Stop"] -> w91
              tunnel: w82 -> [w1992]
              tunnel: w88 -> [w1991]
              tunnel: w75 -> [w1980]
              tunnel: [w1982] -> w81
              tunnel: [w1981] -> w80
              tunnel: w75 -> [w1979]
              tunnel: w75 -> [w1978]
              tunnel: w75 -> [w1977]
              tunnel: ["Set Delay Speed"] -> w79
              tunnel: ["Cycling Bit"] -> w78
              tunnel: ["Test Run Setting"] -> w77
              tunnel: w75 -> [w1972]
              i -> [w1986]
              stop <- w2009 stop-if-true
              n16 = case shown="True" "CP Setting" {
                tunnel: w2010 -> [w2111 w2124]
                tunnel: [w2112 w2118] -> w1994
                tunnel: "VDD" -> [w2099 w2119]
                tunnel: "Select Measurement" -> [w2106 _]
                tunnel: w1992 -> [w2103 w2121]
                tunnel: w1991 -> [w2101 w2123]
                tunnel: [w2102 w2121] -> w1981
                tunnel: [w2101 w2122] -> w1988
                tunnel: [w2099 w2119] -> w1983
                tunnel: w1980 -> [_ w2116]
                tunnel: "Manual Setting" -> [_ w2115]
                frame False {
                  w2100 = 1 items=["Temperature", "Humidity", "TH1", "TH2"] ("Select Measurement")
                  n17 = call "TLTSP_Measurement.vi"("error in (no error)"=w2111, "Select Measurement"=w2106, "VISA resource name"=w2103) -> ("error out"=w2108:errorcluster, "Output"=→"Temp (C)":string, "VISA resource name out"=w2110:refnum<visa-resource-name>)  [unwired: 6 in]
                  n18 = call "Time Delay.vi"("Error In"=w2108, "Delay(ms)"=u32 100) -> ("Error Out"=w2109:errorcluster)  [unwired: 9 in]
                  n19 = call "TLTSP_Measurement.vi"("error in (no error)"=w2109, "Select Measurement"=w2100, "VISA resource name"=w2110) -> ("error out"=w2112:errorcluster, "Output"=→"RH(%)":string, "VISA resource name out"=w2102:refnum<visa-resource-name>)  [unwired: 6 in]
                }
                frame True {
                  n20 = call "E3631A_Voltage Controller updated.vi"("VISA resource name"=w2123, "I_VDD(A)"=0.5, "Channel Controller"=T13."Voltage 1", "Voltage 1"=w2119, "Voltage 2"=3.3, "error in (no error)"=w2124) -> ("VISA resource name out"=w2122:refnum<visa-resource-name>, "error out"=w2117:errorcluster)  [unwired: 8 in]
                  n21 = call "WS1021 CP Setting.vi"("Manual Setting"=w2115, "FPGA"=w2116, "Error In"=w2117) -> ("Error Out"=w2118:errorcluster)  [unwired: 7 in, 1 out]
                }
              }
              n22 = case shown="True" "Initialize ADI" {
                tunnel: w1994 -> [w2081 w2089]
                tunnel: [w2081 w2084] -> w1993
                tunnel: w1988 -> [w2080 w2088]
                tunnel: w1983 -> [_ w2087]
                tunnel: w1979 -> [_ w2083]
                tunnel: [w2080 w2082] -> w1984
                frame False {
                }
                frame True {
                  w2086 = T17 [enum."Voltage 1"] items=["Idle...", "Voltage 1", "Voltage 2", "Voltage 3"]
                  n23 = for {
                    tunnel: w2088 -> [w2096]
                    tunnel: w2087 -> [w2095]
                    tunnel: w2086 -> [w2094] mode=indexing
                    shift-right: [w2092] -> w2085
                    shift-left: w2089 -> [w2098]
                    tunnel: [w2090] -> w2082
                    n24 = call "E3631A_Voltage Controller updated.vi"("VISA resource name"=w2096, "Channel Controller"=w2094, "Voltage 1"=w2095, "Voltage 2"=3.3, "error in (no error)"=w2098) -> ("VISA resource name out"=w2090:refnum<visa-resource-name>, "error out"=w2093:errorcluster)  [unwired: 9 in]
                    n25 = call "Time Delay.vi"("Error In"=w2093, "Delay(ms)"=u32 100) -> ("Error Out"=w2092:errorcluster)  [unwired: 9 in]
                  }
                  n26 = call "WS1021 Initialize AD7747.vi"("Error In"=w2085, "FPGA"=w2083) -> ("Error Out"=w2084:errorcluster)  [unwired: 9 in]
                }
              }
              n27 = case shown="False" "Calibration AD" {
                tunnel: w1993 -> [w2016 w2057]
                tunnel: [w2021 w2052] -> w1987
                tunnel: w1977 -> [w2018 _]
                tunnel: w1986 -> [w2017 _]
                tunnel: w1978 -> [_ w2055]
                tunnel: "DUT Mask Mode (All)" -> [w2014 _]
                tunnel: "DUT Mask Mode (All)" -> [_ w2054]
                tunnel: w1984 -> [w2013 w2051]
                tunnel: w1983 -> [_ w2050]
                tunnel: [w2013 w2047] -> w1982
                tunnel: w1972 -> [w2012 _]
                frame False {
                  n28 = case shown="1, Default" w2017 {
                    tunnel: w2016 -> [w2034 w2039]
                    tunnel: [w2034 w2038] -> w2015
                    tunnel: w2012 -> [_ w2036]
                    frame 0 {
                      w2026 = string[] [] ("Cmin BrdB")
                      w2027 = dbl[] [] ("CMin BrdA")
                      w2029 = string[][] [] ("Brd B_CS VCmin_T0")
                      w2030 = string[][] [] ("Brd B_OS_V3 (fF)")
                      w2028 = string[] [] ("Brd B Delta C%")
                      w2031 = string[][] [] ("Brd B_Beam Cap (fF)")
                      w2032 = string[][] [] ("Data Board A")
                      w2033 = dbl[][] [] ("Board B")
                      n29 = local write "Cmin BrdB"(w2026) -> ()
                      n30 = local write "Cmin BrdA"(w2026) -> ()
                      n31 = local write "Brd A_CS_V1 (fF)"(w2029) -> ()
                      n32 = local write "Brd A_CS_V2 (fF)"(w2029) -> ()
                      n33 = local write "Brd A_CS_V3 (fF)"(w2029) -> ()
                      n34 = local write "Brd B_CS_V1 (fF)"(w2029) -> ()
                      n35 = local write "Brd B_CS_V2 (fF)"(w2029) -> ()
                      n36 = local write "Brd B_CS_V3 (fF)"(w2029) -> ()
                      n37 = local write "Brd B_CS VCmin_T0"(w2029) -> ()
                      n38 = local write "Brd A_CS VCmin_T0"(w2029) -> ()
                      n39 = local write "Brd B_CS VCmin"(w2029) -> ()
                      n40 = local write "Brd A_CS VCmin"(w2029) -> ()
                      n41 = local write "Brd B_OS_V3 (fF)"(w2030) -> ()
                      n42 = local write "Brd B_OS_V2 (fF)"(w2030) -> ()
                      n43 = local write "Brd B_OS_V1 (fF)"(w2030) -> ()
                      n44 = local write "Brd A_OS_V3 (fF)"(w2030) -> ()
                      n45 = local write "Brd A_OS_V1 (fF)"(w2030) -> ()
                      n46 = local write "Brd A_OS_V2 (fF)"(w2030) -> ()
                      n47 = local write "Brd B_Beam Cap (fF)"(w2031) -> ()
                      n48 = local write "Brd A_Beam Cap (fF)"(w2031) -> ()
                      n49 = local write "Brd B_VPI Cap (fF)"(w2031) -> ()
                      n50 = local write "Brd A_VPI Cap (fF)"(w2031) -> ()
                      n51 = local write "Brd B Delta C%"(w2028) -> ()
                      n52 = local write "Brd A Delta C%"(w2028) -> ()
                      n53 = local write "VPI Brd B Delta C%"(w2028) -> ()
                      n54 = local write "VPI Brd A Delta C%"(w2028) -> ()
                      n55 = local write "IDD Measurement(uA)"(w2028) -> ()
                      n56 = local write "CMin BrdA (fF)"(w2027) -> ()
                      n57 = local write "CMin BrdB (fF)"(w2027) -> ()
                      n58 = local write "Data Board A"(w2032) -> ()
                      n59 = local write "Data Board B"(w2032) -> ()
                      n60 = local write "Board B"(w2033) -> ()
                      n61 = local write "Board A"(w2033) -> ()
                    }
                    frame 1, Default {
                      n62 = case shown="True" "Verify Beams" {
                        tunnel: w2039 -> [w2041 w2046]
                        tunnel: [w2041 w2045] -> w2038
                        tunnel: w2036 -> [_ w2044]
                        tunnel: "Manual Command" -> [_ w2042]
                        frame False {
                        }
                        frame True {
                          n63 = call "WSVCAP SHL Host TL RFFE Write - Multiple DUTs - Common Data.vi"("Data Out"=w2042, "error in"=w2046, "FPGA"=w2044, "Log (T)"=FALSE) -> ("error out"=w2045:errorcluster)  [unwired: 11 in]
                        }
                      }
                      n64 = local write "Status"("Idle...." ("Status")) -> ()
                    }
                  }
                  n65 = call "WS1021 ADI Read 64 DUT.vi"("DUT Mask Mode (All)"=w2014, "FPGA"=w2018, "Error In"=w2015) -> ("Error Out"=w2020:errorcluster, "AD7747 Values"=w2019:string[][])  [unwired: 7 in]
                  n66 = call "WS1021 I2C Monitor Single Board.vi"("SN Brd B"="SN Brd B", "SN Brd A"="SN Brd A", "Error In"=w2020, "AD7747 Values"=w2019) -> ("Error Out"=w2021:errorcluster, "I2C Board B"=→"AD7747 Value Brd B":string[][], "I2C Board A"=→"AD7747 Value Brd A":string[][])  [unwired: 5 in]
                }
                frame True {
                  n67 = flat-sequence {
                    tunnel: w2057 -> [w2063]
                    tunnel: [w2062] -> w2056
                    tunnel: w2051 -> [w2061]
                    tunnel: w2050 -> [w2060]
                    tunnel: [w2058] -> w2049
                    tunnel: w2056 -> [w2073]
                    tunnel: w2055 -> [w2067]
                    tunnel: w2054 -> [w2068]
                    tunnel: [w2066] -> w2053
                    tunnel: w2049 -> [w2065]
                    tunnel: [w2065] -> w2048
                    tunnel: w2053 -> [w2079]
                    tunnel: [w2078] -> w2052
                    tunnel: w2048 -> [w2077]
                    tunnel: [w2074] -> w2047
                    frame #0 {
                      # "Set Voltage"
                      n68 = call "E3631A_Voltage Controller updated.vi"("VISA resource name"=w2061, "Channel Controller"=T13."Voltage 1", "Voltage 1"=w2060, "error in (no error)"=w2063) -> ("VISA resource name out"=w2058:refnum<visa-resource-name>, "error out"=w2062:errorcluster)  [unwired: 10 in]
                      n69 = One Button Dialog(message="Please verify all DUTs are empty...") -> ()  [unwired: 1 in, 1 out]
                    }
                    frame #1 {
                      # "Set ADI"
                      n70 = call "WS1021 ADI CAPDAC Setting.vi"("DUT Mask Mode (All)"=w2068, "FPGA"=w2067, "Error In"=w2073, "CAPDAC Value"="CAPDAC Value") -> ("Error Out"=w2071:errorcluster)  [unwired: 7 in]
                      n71 = call "WS1021 ADI OFFSET CAL.vi"("DUT Mask Mode (All)"=w2068, "FPGA"=w2067, "Error In"=w2071) -> ("Error Out"=w2070:errorcluster)  [unwired: 8 in]
                      n72 = call "Time Delay.vi"("Error In"=w2070, "Delay(ms)"=u32 100) -> ("Error Out"=w2066:errorcluster)  [unwired: 9 in]
                    }
                    frame #2 {
                      # "Set Voltage"
                      n73 = call "E3631A_Voltage Controller updated.vi"("VISA resource name"=w2077, "Channel Controller"=T13."Voltage 1", "Voltage 1"=0.0, "error in (no error)"=w2079) -> ("VISA resource name out"=w2074:refnum<visa-resource-name>, "error out"=w2078:errorcluster)  [unwired: 10 in]
                    }
                  }
                }
              }
              n74 = call "Time_stamp.vi"() -> ("date/time string"=w2006:string, "date string"=w2007:string)  [unwired: 2 in]
              "Current Time" <- w2006
              "Current Date" <- w2007
              n75 = call "Time Delay.vi"("Error In"=w1987, "Delay(ms)"=u32 250) -> ("Error Out"=w1990:errorcluster)  [unwired: 9 in]
              n76 = Equal?(x=w2007, y="Start Date") -> (x = y?=w2003:bool)
              n77 = Equal?(x=w2006, y="Start Time") -> (x = y?=w2002:bool)
              n78 = And(x=w2003, y=w2002) -> (x .and. y?=w2001:bool)
              n79 = Unbundle By Name(w1990) -> ("status"=w2008:bool)
              n80 = Compound Arithmetic op=OR(w2008, w2001, "Start", "Stop") -> (w2009:bool)
              "Test Run Selected" <- "Test Run Setting"
            }
            n81 = case shown="False" w91 {
              tunnel: w94 -> [w120 w1971]
              tunnel: [w164 w1971] -> w92
              tunnel: w90 -> [w149 w1970]
              tunnel: w89 -> [w145 w1969]
              tunnel: w81 -> [w148 w1968]
              tunnel: w80 -> [w143 w1967]
              tunnel: [w147 w1968] -> w87
              tunnel: [w146 w1970] -> w86
              tunnel: [w144 w1969] -> w85
              tunnel: [w142 w1967] -> w84
              tunnel: w83 -> [w122 _]
              tunnel: w75 -> [w104 _]
              tunnel: w75 -> [w101 _]
              tunnel: w79 -> [w97 _]
              tunnel: w78 -> [w96 _]
              tunnel: w77 -> [w95 _]
              frame False {
                n82 = call "WS1021 Individual Beam Controls.vi"("Error In"=w120, "USID"="07") -> ("Error Out"=w119:errorcluster, "Reg 2 Cmd"=w113:string[], "Reg 3 Cmd"=w114:string[], "Reg 2 Name"=w115:string[], "VPI_Cmd"=w112:string[], "Reg 3 Name"=w116:string[], "VPI_Name"=w117:string[])  [unwired: 3 in]
                n83 = Unbundle By Name(w95) -> ("OTP ?"=w155:bool, "STRESS ?"=w154:bool, "VPI ?"=w153:bool, "OPEN STATE VCMIN ?"=w152:bool, "CLOSE STATE VCMIN ?"=w151:bool, "RPM (Verify Socket) ?"=w150:bool, "HS CHK?"=w132:bool)
                n84 = Unbundle By Name("Info Brd B") -> ("Lot #"=w139:string, "Wafer #"=w138:string, "Board"=w137:string, "Comment"=w136:string, "File Name"=w135:string, "Data File Path Control"=w134:path)
                n85 = Unbundle By Name("Info Brd A") -> ("Lot #"=w161:string, "Wafer #"=w160:string, "Board"=w159:string, "Comment"=w158:string, "File Name"=w157:string, "Data File Path Control"=w156:path)
                n86 = Unbundle By Name("Test Condition Setting") -> ("Freq (KHz)"=w130:string, "ACV (V)"=w129:string, "AC Freq (Hz)"=w128:string, "Temp (C)"=w127:string, "DCV (V)"=w126:dbl, "CYC RP (x1000)"=w125:u64, "HD RP (Min)"=w124:u64, "RPM Delay (s)"=w123:u64, "Select VCmin"=w105:u16)
                n87 = while {
                  tunnel: w119 -> [w241]
                  tunnel: [w171] -> w164
                  tunnel: w155 -> [w239]
                  tunnel: w154 -> [w238]
                  tunnel: w153 -> [w237]
                  tunnel: w152 -> [w236]
                  tunnel: w151 -> [w235]
                  tunnel: w150 -> [w234]
                  tunnel: w161 -> [w233]
                  tunnel: w160 -> [w232]
                  tunnel: w159 -> [w231]
                  tunnel: w158 -> [w230]
                  tunnel: w157 -> [w229]
                  tunnel: "Test Program" -> [w228]
                  tunnel: w130 -> [w227]
                  tunnel: w129 -> [w226]
                  tunnel: w128 -> [w225]
                  tunnel: w127 -> [w224]
                  tunnel: w125 -> [w223]
                  tunnel: w123 -> [w222]
                  tunnel: w156 -> [w221]
                  tunnel: w149 -> [w220]
                  tunnel: w148 -> [w219]
                  tunnel: [w218] -> w147
                  tunnel: [w217] -> w146
                  tunnel: w145 -> [w216]
                  tunnel: [w215] -> w144
                  tunnel: w143 -> [w214]
                  tunnel: [w213] -> w142
                  tunnel: string[][] [] -> [w212]
                  tunnel: w139 -> [w211]
                  tunnel: w138 -> [w210]
                  tunnel: w137 -> [w209]
                  tunnel: w136 -> [w208]
                  tunnel: w135 -> [w207]
                  tunnel: w134 -> [w206]
                  tunnel: string[][] [] -> [w205]
                  tunnel: w132 -> [w204]
                  tunnel: w126 -> [w203]
                  tunnel: w124 -> [w202]
                  tunnel: w122 -> [w201]
                  shift-right: [w197] -> _
                  shift-left: u64 0 -> [w198]
                  tunnel: w117 -> [w194]
                  tunnel: w116 -> [w193]
                  tunnel: w115 -> [w192]
                  tunnel: w114 -> [w191]
                  tunnel: w113 -> [w190]
                  tunnel: w112 -> [w189]
                  tunnel: "Select CP Stress" -> [w188]
                  tunnel: "Data Brd B?" -> [w187]
                  tunnel: "Data Brd A?" -> [w186]
                  tunnel: "OS_Voltage(V)" -> [w185]
                  tunnel: "CS_Voltage(V)" -> [w184]
                  tunnel: w105 -> [w183]
                  tunnel: w104 -> [w182]
                  tunnel: "CP Measurement" -> [w181]
                  tunnel: "Select CP VPI" -> [w180]
                  tunnel: w101 -> [w179]
                  tunnel: "Clock Rate Cycle(Hz)" -> [w176]
                  tunnel: "RFFE Slave Address" -> [w175]
                  tunnel: "Clock Rate Meas(Hz)" -> [w174]
                  tunnel: w97 -> [w173]
                  tunnel: w96 -> [w172]
                  i -> [w200]
                  stop <- w169 stop-if-true
                  # "Read Points"
                  n88 = local read "SN Brd B"() -> (w177:string[])
                  n89 = Index Array(array=w201, index (row)=w200, index (col)=0 ("disabled index (col)")) -> (element=w195:dbl)
                  n90 = local read "SN Brd A"() -> (w178:string[])
                  n91 = To Unsigned Quad Integer(1:w195) -> (0:w196:u64)
                  n92 = while {
                    tunnel: w241 -> [w321]
                    tunnel: [w298] -> w168
                    shift-right: [w306] -> _
                    shift-left: Test_Sequences."VDD" ("Test Sequences") -> [w320]
                    tunnel: w239 -> [w319]
                    tunnel: w238 -> [w318]
                    tunnel: w237 -> [w317]
                    tunnel: w236 -> [w316]
                    tunnel: w235 -> [w315]
                    tunnel: w234 -> [w314]
                    tunnel: w233 -> [w313]
                    tunnel: w232 -> [w312]
                    tunnel: w231 -> [w311]
                    tunnel: w230 -> [w310]
                    tunnel: w229 -> [w309]
                    tunnel: w221 -> [w308]
                    tunnel: w228 -> [w307]
                    tunnel: w227 -> [w305]
                    tunnel: w226 -> [w304]
                    tunnel: w225 -> [w303]
                    tunnel: w224 -> [w302]
                    tunnel: w223 -> [w301]
                    tunnel: w202 -> [w300]
                    tunnel: w222 -> [w299]
                    tunnel: w220 -> [w296]
                    tunnel: w219 -> [w295]
                    tunnel: [w294] -> w218
                    tunnel: [w293] -> w217
                    tunnel: w216 -> [w292]
                    tunnel: [w291] -> w215
                    tunnel: w214 -> [w290]
                    tunnel: [w289] -> w213
                    tunnel: [w246] -> w167
                    tunnel: w200 -> [w285]
                    shift-right: [w247] -> _
                    shift-left: w212 -> [w284]
                    tunnel: w211 -> [w283]
                    tunnel: w210 -> [w282]
                    tunnel: w209 -> [w281]
                    tunnel: w208 -> [w280]
                    tunnel: w207 -> [w279]
                    tunnel: w206 -> [w278]
                    shift-right: [w248] -> _
                    shift-left: w205 -> [w277]
                    tunnel: w204 -> [w276]
                    tunnel: w203 -> [w275]
                    tunnel: w196 -> [w274]
                    tunnel: w198 -> [w273]
                    tunnel: [w272] -> w197
                    tunnel: w194 -> [w271]
                    tunnel: w193 -> [w270]
                    tunnel: w192 -> [w269]
                    tunnel: w191 -> [w268]
                    tunnel: w190 -> [w267]
                    tunnel: w189 -> [w266]
                    tunnel: w188 -> [w265]
                    tunnel: w187 -> [w264]
                    tunnel: w186 -> [w263]
                    tunnel: w185 -> [w262]
                    tunnel: w184 -> [w261]
                    tunnel: w183 -> [w260]
                    tunnel: w182 -> [w259]
                    tunnel: w181 -> [w258]
                    tunnel: w180 -> [w257]
                    tunnel: w179 -> [w256]
                    tunnel: w178 -> [w255]
                    tunnel: w177 -> [w254]
                    tunnel: w176 -> [w253]
                    tunnel: w175 -> [w252]
                    tunnel: w174 -> [w251]
                    tunnel: w173 -> [w250]
                    tunnel: w172 -> [w249]
                    tunnel: [w245] -> w166
                    shift-right: [w243] -> _
                    shift-left: "" -> [w242]
                    stop <- w288 stop-if-true
                    # "Measurement"
                    n93 = case shown="\"Stress\"" w320 {
                      selector: w320 -> [w338 w444 w551 w726 _ _ _ _ _ _ _]
                      tunnel: w321 -> [w367 w458 w577 w750 w1046 w1144 w1279 w1417 w1553 w1803 w1904]
                      tunnel: [w377 w461 w589 w752 w1055 w1179 w1285 w1424 w1571 w1815 w1881] -> w286
                      tunnel: [w376 w460 w590 w753 w1056 w1180 w1284 w1423 w1572 w1814 _] -> w306
                      tunnel: w319 -> [_ w459 _ w747 _ _ _ _ _ _ _]
                      tunnel: w318 -> [_ _ _ w748 _ _ _ _ _ _ _]
                      tunnel: w317 -> [_ _ _ _ _ _ w1275 _ _ _ _]
                      tunnel: w316 -> [_ _ _ _ _ _ _ w1418 _ _ _]
                      tunnel: w315 -> [_ _ _ _ _ _ _ _ w1536 _ _]
                      tunnel: w314 -> [_ _ _ w751 _ _ _ _ _ _ _]
                      tunnel: w313 -> [w369 _ w549 _ _ _ _ _ _ _ w1899]
                      tunnel: w312 -> [w368 _ w548 _ _ _ _ _ _ _ w1898]
                      tunnel: w311 -> [w355 _ _ _ _ _ _ _ _ _ _]
                      tunnel: w310 -> [_ _ _ _ _ _ _ _ _ w1797 _]
                      tunnel: w309 -> [_ _ w530 _ _ _ _ _ _ w1788 w1897]
                      tunnel: w308 -> [_ _ w550 _ _ _ _ _ _ w1794 w1879]
                      tunnel: w307 -> [_ _ _ _ _ _ _ _ _ w1800 _]
                      tunnel: w305 -> [_ _ w571 _ _ _ _ _ _ _ _]
                      tunnel: w304 -> [_ _ w572 _ _ _ _ _ _ _ _]
                      tunnel: w303 -> [_ _ w573 _ _ _ _ _ _ _ _]
                      tunnel: w302 -> [_ _ w574 _ _ _ _ _ _ _ _]
                      tunnel: w301 -> [_ _ _ w728 _ _ _ _ _ _ _]
                      tunnel: w300 -> [_ _ _ w739 _ _ _ _ _ _ _]
                      tunnel: w299 -> [_ _ _ w745 _ _ _ _ _ _ _]
                      tunnel: w296 -> [w341 w451 w584 w715 w1054 w1178 w1282 w1416 w1566 w1813 w1896]
                      tunnel: w295 -> [w350 w449 w580 w743 w1049 w1176 w1280 w1420 w1569 w1811 w1895]
                      tunnel: [w343 w449 w579 w743 w1049 w1176 w1280 w1420 w1569 w1811 w1894] -> w294
                      tunnel: [w341 w451 w583 w713 w1054 w1178 w1282 w1409 w1562 w1813 w1893] -> w293
                      tunnel: w292 -> [w342 w450 w582 w744 w1044 w1177 w1281 w1421 w1570 w1812 w1892]
                      tunnel: [w342 w450 w581 w744 w1043 w1177 w1281 w1421 w1570 w1812 w1892] -> w291
                      tunnel: w290 -> [w340 w448 w563 w742 w1048 w1174 w1283 w1419 w1568 w1810 w1891]
                      tunnel: [w340 w448 w558 w742 w1048 w1174 w1283 w1419 w1568 w1810 w1891] -> w289
                      tunnel: [w332 w432 w540 w706 w1029 w1137 w1255 w1389 w1537 w1786 TRUE ("true")] -> w287
                      tunnel: w285 -> [w352 _ _ w746 _ w1149 _ _ w1549 _ _]
                      tunnel: w284 -> [w370 w453 w586 w740 w1050 w1165 w1272 w1413 w1558 w1778 _]
                      tunnel: w283 -> [w363 _ w544 _ _ _ _ _ _ _ w1878]
                      tunnel: w282 -> [w362 _ w543 _ _ _ _ _ _ _ w1877]
                      tunnel: w281 -> [w361 _ _ _ _ _ _ _ _ _ _]
                      tunnel: w280 -> [_ _ _ _ _ _ _ _ _ w1799 _]
                      tunnel: w279 -> [_ _ w531 _ _ _ _ _ _ w1787 w1875]
                      tunnel: w278 -> [_ _ w546 _ _ _ _ _ _ w1795 _]
                      tunnel: w277 -> [w360 w455 w588 w741 w1053 w1167 w1273 w1414 w1560 w1777 _]
                      tunnel: [w357 w454 w587 w732 w1052 w1166 w1274 w1411 w1559 _ _] -> w248
                      tunnel: [w356 w452 w585 w731 w1051 w1164 w1271 w1412 w1557 _ _] -> w247
                      tunnel: w276 -> [_ _ w578 _ _ _ _ _ _ _ _]
                      tunnel: w275 -> [_ _ _ w725 _ _ _ _ _ _ _]
                      tunnel: w274 -> [_ _ _ w729 _ _ _ _ _ _ _]
                      tunnel: w273 -> [w339 w447 w552 w738 w1047 w1175 w1276 w1422 w1567 w1809 _]
                      tunnel: [w339 w447 w552 w735 w1047 w1175 w1276 w1422 w1567 w1809 w1889] -> w272
                      tunnel: w271 -> [_ _ _ _ _ _ w1278 _ _ w1789 _]
                      tunnel: w270 -> [_ _ _ _ _ w1170 _ _ _ w1791 _]
                      tunnel: w269 -> [_ _ _ _ _ w1169 _ _ _ w1790 _]
                      tunnel: w268 -> [_ _ _ _ _ w1173 _ _ _ _ _]
                      tunnel: w267 -> [_ _ _ _ _ w1172 _ _ _ _ _]
                      tunnel: w266 -> [_ _ _ _ _ _ w1277 _ _ _ _]
                      tunnel: w265 -> [_ w445 _ _ _ _ _ _ _ _ _]
                      tunnel: w264 -> [_ _ w537 _ w1025 w1135 w1247 w1382 w1526 w1774 w1880]
                      tunnel: w263 -> [_ _ w536 _ w1023 w1134 w1248 w1381 w1525 w1775 w1884]
                      tunnel: w262 -> [_ _ _ _ _ _ _ w1415 _ _ _]
                      tunnel: w261 -> [_ _ _ _ _ _ _ _ w1565 _ _]
                      tunnel: w260 -> [_ _ _ _ _ _ _ _ _ _ _]
                      tunnel: w259 -> [w326 w443 w547 w704 w1037 w1138 w1268 w1390 w1530 _ _]
                      tunnel: w258 -> [_ _ _ _ _ w1139 _ _ w1533 _ _]
                      tunnel: w257 -> [_ _ _ _ _ _ w1269 _ _ _ _]
                      tunnel: w256 -> [_ _ _ _ _ w1140 w1270 _ w1534 _ _]
                      tunnel: w255 -> [w333 _ w541 _ _ _ _ _ _ _ _]
                      tunnel: w254 -> [w335 _ w542 _ _ _ _ _ _ _ _]
                      tunnel: w253 -> [_ _ _ w711 _ _ _ _ _ _ _]
                      tunnel: w252 -> [w327 _ _ w712 _ _ _ _ _ _ _]
                      tunnel: w251 -> [w328 _ _ w710 _ _ _ _ _ _ _]
                      tunnel: w250 -> [_ _ _ w709 _ _ _ _ _ _ _]
                      tunnel: w249 -> [_ _ _ w708 _ _ _ _ _ _ _]
                      tunnel: [w332 w432 w540 FALSE ("true") w1029 w1137 w1255 w1389 w1537 w1786 w1887] -> w246
                      tunnel: [w332 w432 w540 w706 w1029 w1137 w1255 w1389 w1537 w1786 FALSE ("true")] -> w245
                      tunnel: [w322 w431 w532 "" w1028 w1136 w1250 w1384 w1527 w1773 ""] -> w244
                      tunnel: w242 -> [_ _ _ _ _ _ _ _ _ _ w1876]
                      frame "VDD" {
                        w331 = string[][] [] ("Data Board B")
                        w332 = FALSE ("true")
                        n94 = Get Date/Time In Seconds() -> (seconds since 1Jan1904=w374:timestamp)
                        n95 = Format Into String(format string="%s", w338) -> (resulting string=w336:string)  [unwired: 2 in, 1 out]
                        n96 = local read "VDD"() -> (w349:dbl)
                        n97 = Get Date/Time String(seconds (now)=w374, want seconds? (F)=TRUE) -> (date string=w372:string, time string=w371:string)  [unwired: 1 in]
                        n98 = local write "Status"(w336) -> ()
                        n99 = for {
                          N: 32 -> [_]
                          tunnel: w372 -> [w407]
                          tunnel: w371 -> [w406]
                          tunnel: [w407] -> w345 mode=indexing
                          tunnel: [w406] -> w344 mode=indexing
                          tunnel: w369 -> [w404]
                          tunnel: w368 -> [w403]
                          shift-right: [w405] -> w351
                          shift-left: w367 -> [w405]
                          tunnel: [w397] -> w364 mode=indexing
                          tunnel: [w404] -> w366 mode=indexing
                          tunnel: [w403] -> w365 mode=indexing
                          tunnel: w363 -> [w402]
                          tunnel: [w402] -> w359 mode=indexing
                          tunnel: w362 -> [w401]
                          tunnel: [w401] -> w358 mode=indexing
                          tunnel: [w400] -> w353 mode=indexing
                          tunnel: w361 -> [w400]
                          tunnel: [w399] -> w354 mode=indexing
                          tunnel: w355 -> [w399]
                          tunnel: w335 -> [w398] mode=indexing
                          tunnel: [w398] -> w334 mode=indexing
                          tunnel: w333 -> [w397] mode=indexing
                        }
                        n100 = case shown="0" w352 {
                          tunnel: w351 -> [w394 w395]
                          tunnel: [w386 w395] -> w346
                          tunnel: w349 -> [w390 _]
                          tunnel: w350 -> [w389 w396]
                          tunnel: [w388 w396] -> w343
                          frame 0 {
                            w387 = string[] [] ("Brd A Delta C%")
                            w391 = 1 items=["Channel 1"=1, "Channel 2"=2, "Channel 3"=3] ("Channel (1: Channel 1)")
                            n101 = call "E3631A Configuration Output.vi"("Channel (1: Channel 1)"=w391, "error in (no error)"=w394, "Voltage Level (0.0 V)"=w390, "VISA resource name"=w389) -> ("error out"=w393:errorcluster, "VISA resource name out"=w388:refnum<visa-resource-name>)  [unwired: 6 in]
                            n102 = call "Time Delay.vi"("Error In"=w393, "Delay(ms)"=u32 100) -> ("Error Out"=w386:errorcluster)  [unwired: 9 in]
                            n103 = local write "VPI Brd A Delta C%"(w387) -> ()
                            n104 = local write "VPI Brd B Delta C%"(w387) -> ()
                            n105 = local write "T0_Brd A Delta C%"(w387) -> ()
                            n106 = local write "T0_Brd B Delta C%"(w387) -> ()
                          }
                          frame 1, Default {
                          }
                        }
                        n107 = local write "Data Board A"(w331) -> ()
                        n108 = local write "Data Board B"(w331) -> ()
                        n109 = for {
                          N: 32 -> [_]
                          tunnel: w349 -> [w385]
                          tunnel: [w383] -> w347 mode=indexing
                          shift-right: [w382] -> w329
                          shift-left: w346 -> [w382]
                          n110 = Number To Fractional String(number=w385, precision (6)=i16 2) -> (F-format string=w383:string)  [unwired: 2 in]
                        }
                        n111 = call "WSVCAP SHL Host TL RFFE Configure.vi"("RFFE Slave Address"=w327, "Clock Rate (Hz)"=w328, "error in"=w329, "Log (T)"=FALSE, "FPGA"=w326) -> ("error out"=w325:errorcluster)  [unwired: 9 in, 1 out]
                        n112 = case shown="Error" w325 {
                          selector: w325 -> [w379 _]
                          tunnel: [w379 errorcluster {"status"=FALSE, "code"=0, "source"=""} ("Error Out")] -> w324
                          tunnel: ["0" "1"] -> w323
                          frame No Error {
                          }
                          frame Error {
                          }
                        }
                        n113 = flat-sequence {
                          tunnel: w324 -> [w428]
                          tunnel: [w428] -> w377
                          tunnel: [w427] -> w376
                          tunnel: w370 -> [w426]
                          tunnel: w345 -> [w422]
                          tunnel: w344 -> [w421]
                          tunnel: w366 -> [w425]
                          tunnel: w365 -> [w424]
                          tunnel: w364 -> [w416]
                          tunnel: w360 -> [w423]
                          tunnel: w359 -> [w420]
                          tunnel: w358 -> [w419]
                          tunnel: w334 -> [w414]
                          tunnel: [w418] -> w357
                          tunnel: [w417] -> w356
                          tunnel: w354 -> [w415]
                          tunnel: w353 -> [w413]
                          tunnel: w347 -> [w412]
                          tunnel: w347 -> [w411]
                          tunnel: w345 -> [w410]
                          tunnel: w344 -> [w409]
                          tunnel: w323 -> [w408]
                          tunnel: [w408] -> w322
                          frame #0 {
                            n114 = Build Array (concatenate)(w423, w410, w409, w420, w419, w413, w414, w411) -> (w418:string[][])
                            n115 = Build Array (concatenate)(w426, w422, w421, w425, w424, w415, w416, w412) -> (w417:string[][])
                            n116 = Select(t=Test_Sequences."Save Data" ("Test Sequences"), s=w428, f=Test_Sequences."CP Setting" ("Test Sequences")) -> (s? t:f=w427:T8)
                          }
                        }
                      }
                      frame "CP Setting" {
                        w432 = FALSE ("true")
                        n117 = flat-sequence {
                          tunnel: w458 -> [w504]
                          tunnel: [w506] -> w457
                          tunnel: [w502] -> w435
                          tunnel: w445 -> [w503]
                          tunnel: w444 -> [w501]
                          tunnel: w443 -> [w495]
                          tunnel: [w488] -> w437
                          frame #0 {
                            w494 = T18 0 items=["both", "start of string", "end of string"] ("location (both)")
                            # "Set CP For Stressing"
                            n118 = call "WS1021 CP Voltages Setting.vi"("Select CPV"=w503, "Error In"=w504) -> ("Error Out"=w498:errorcluster, "CP Select"=w496:string, "Cmd Send out"=w486:string)  [unwired: 4 in, 3 out]
                            n119 = Build Array (concatenate)(string[] ["074000", "074080", "074101"], w486) -> (w485:string[])
                            n120 = for {
                              tunnel: w495 -> [w512]
                              shift-right: [w511] -> w497
                              shift-left: w498 -> [w513]
                              tunnel: w485 -> [w507] mode=indexing
                              n121 = call "WSVCAP SHL Host TL RFFE Write - Multiple DUTs - Common Data.vi"("Data Out"=w507, "error in"=w513, "FPGA"=w512, "Log (T)"=FALSE) -> ("error out"=w510:errorcluster)  [unwired: 11 in]
                              n122 = call "Time Delay.vi"("Error In"=w510, "Delay(ms)"=u32 25) -> ("Error Out"=w511:errorcluster)  [unwired: 9 in]
                            }
                            n123 = call <vilib>:"Trim Whitespace.vi"("string"=w486, "location (both)"=w494) -> ("trimmed string"=w490:string)
                            n124 = String Length(string=w490) -> (length=w493:i32)
                            n125 = Subtract(x=w493, y=2) -> (x-y=w491:i32)
                            n126 = String Subset(string=w490, offset (0)=w491) -> (substring=w489:string)  [unwired: 1 in]
                            n127 = Format Into String(format string="%s", w501) -> (resulting string=w499:string)  [unwired: 2 in, 1 out]
                            n128 = for {
                              N: 32 -> [_]
                              shift-right: [w516] -> w506
                              shift-left: w497 -> [w516]
                              tunnel: w496 -> [w515]
                              tunnel: [w515] -> w502 mode=indexing
                              tunnel: w489 -> [w514]
                              tunnel: [w514] -> w488 mode=indexing
                            }
                            n129 = local write "Status"(w499) -> ()
                          }
                        }
                        n130 = case shown="True" w459 {
                          tunnel: w457 -> [w476 w482]
                          tunnel: [w475 w481] -> w456
                          tunnel: [w473 w480] -> w446
                          frame False {
                            # "CP CYC, NO OTP"
                            n131 = for {
                              N: 32 -> [_]
                              shift-right: [w478] -> w475
                              shift-left: w476 -> [w478]
                              tunnel: ["N"] -> w473 mode=indexing
                            }
                          }
                          frame True {
                            # "CP CYC, OTP"
                            n132 = for {
                              N: 32 -> [_]
                              shift-right: [w484] -> w481
                              shift-left: w482 -> [w484]
                              tunnel: ["Y"] -> w480 mode=indexing
                            }
                          }
                        }
                        n133 = call "WSVCAP SHL Host TL RFFE Read - Multiple DUTs - Common Data.vi"("Data Out"="076C", "error in"=w456, "FPGA"=w443, "Log (T)"=FALSE) -> ("RFFE Data In"=w436:string[], "error out"=w441:errorcluster)  [unwired: 10 in]
                        n134 = call "Time Delay.vi"("Error In"=w441, "Delay(ms)"=u32 10) -> ("Error Out"=w438:errorcluster)  [unwired: 9 in]
                        n135 = for {
                          tunnel: w437 -> [w468] mode=indexing
                          tunnel: w436 -> [w467] mode=indexing
                          shift-right: [w464] -> w433
                          shift-left: w438 -> [w465]
                          tunnel: w435 -> [w463] mode=indexing
                          tunnel: [w462] -> w434 mode=indexing
                          n136 = Equal?(x=w468, y=w467) -> (x = y?=w466:bool)
                          n137 = case shown="True" w466 {
                            tunnel: w465 -> [w469 w472]
                            tunnel: [w469 w472] -> w464
                            tunnel: w463 -> [_ w471]
                            tunnel: ["F" ("CP Select") w471] -> w462
                            frame False {
                            }
                            frame True {
                            }
                          }
                        }
                        "Verify CP Stress" <- w434
                        n138 = flat-sequence {
                          tunnel: w433 -> [w527]
                          tunnel: [w527] -> w461
                          tunnel: [w526] -> w460
                          tunnel: w455 -> [w525]
                          tunnel: [w524] -> w454
                          tunnel: w453 -> [w523]
                          tunnel: [w522] -> w452
                          tunnel: w435 -> [w521]
                          tunnel: w435 -> [w520]
                          tunnel: w446 -> [w518]
                          tunnel: w446 -> [w519]
                          tunnel: [""] -> w431
                          frame #0 {
                            n139 = Build Array (concatenate)(w525, w520, w519) -> (w524:string[][])
                            n140 = Build Array (concatenate)(w523, w521, w518) -> (w522:string[][])
                            n141 = Select(t=Test_Sequences."Save Data" ("Test Sequences"), s=w527, f=Test_Sequences."HS CHK" ("Test Sequences")) -> (s? t:f=w526:T8)
                          }
                        }
                      }
                      frame "HS CHK" {
                        w560 = 1 items=["Temperature", "Humidity", "TH1", "TH2"] ("Select Measurement")
                        w561 = 0 items=["Temperature", "Humidity", "TH1", "TH2"] ("Select Measurement")
                        w540 = FALSE ("true")
                        n142 = case shown="False" w578 {
                          tunnel: w577 -> [w606 w626]
                          tunnel: [w605 w615] -> w564
                          tunnel: [w604 w630] -> w576
                          tunnel: w551 -> [_ w633]
                          tunnel: w550 -> [_ w629]
                          tunnel: w549 -> [_ w628]
                          tunnel: w548 -> [_ w627]
                          tunnel: w547 -> [_ w620]
                          tunnel: w546 -> [_ w625]
                          tunnel: [w603 w624] -> w545
                          tunnel: w544 -> [_ w622]
                          tunnel: w543 -> [_ w621]
                          tunnel: w542 -> [_ w619]
                          tunnel: w541 -> [_ w618]
                          tunnel: [w602 w617] -> w539
                          tunnel: [w602 w614] -> w538
                          tunnel: w537 -> [_ w613]
                          tunnel: w536 -> [_ w612]
                          tunnel: w531 -> [_ w611]
                          tunnel: w530 -> [_ w610]
                          frame False {
                            w602 = bool[] []
                            n143 = for {
                              N: 32 -> [_]
                              shift-right: [w609] -> w605
                              shift-left: w606 -> [w609]
                              tunnel: [w608] -> w604 mode=indexing
                              tunnel: [w608] -> w603 mode=indexing
                              w608 = "0"
                            }
                          }
                          frame True {
                            w623 = string[] ["01", "02", "04", "08", "03", "06", "0C", "07", "0E", "0F", "07", "03", "00"] ("HS CHK CNTRL")
                            n144 = case shown="True" w612 {
                              tunnel: [w634 w655] -> w630
                              tunnel: w629 -> [_ w653]
                              tunnel: w628 -> [_ w651]
                              tunnel: w627 -> [_ w650]
                              tunnel: w626 -> [w638 w649]
                              tunnel: w623 -> [_ w648]
                              tunnel: w620 -> [_ w647]
                              tunnel: w618 -> [_ w646]
                              tunnel: [bool[] [] ("Pass/Fail?") w645] -> w617
                              tunnel: [w637 w642] -> w616
                              tunnel: w610 -> [_ w641]
                              frame False {
                                n145 = for {
                                N: 32 -> [_]
                                shift-right: [w640] -> w637
                                shift-left: w638 -> [w640]
                                tunnel: [""] -> w634 mode=indexing
                                }
                              }
                              frame True {
                                w644 = TRUE ("Start")
                                n146 = call "WS1021 RFFE Multi Dut Handshake Check.vi"("HS CHK CNTRL"=w648, "TMN DC\\CAP Data Log File Path"=w653, "Debug?"=FALSE, "Set Register"="3", "Select Brd"=enum16{"A", "B"}."A", "Lot#"=w651, "Stop Button"=w644, "Wafer #"=w650, "File Name"=w641, "Error In"=w649, "FPGA"=w647, "SN#"=w646, "Start"=w644) -> ("Status"=w655:string[], "Pass/Fail?"=w645:bool[], "Error Out"=w642:errorcluster)
                              }
                            }
                            n147 = Format Into String(format string="%s", w633) -> (resulting string=w631:string)  [unwired: 2 in, 1 out]
                            n148 = local write "Status"(w631) -> ()
                            n149 = case shown="True" w613 {
                              tunnel: w625 -> [_ w677]
                              tunnel: [w656 w676] -> w624
                              tunnel: w623 -> [_ w675]
                              tunnel: w622 -> [_ w673]
                              tunnel: w621 -> [_ w672]
                              tunnel: w620 -> [_ w671]
                              tunnel: w619 -> [_ w670]
                              tunnel: w616 -> [w660 w666]
                              tunnel: [w659 w665] -> w615
                              tunnel: [bool[] [] ("Pass/Fail?") w664] -> w614
                              tunnel: w611 -> [_ w663]
                              frame False {
                                n150 = for {
                                N: 32 -> [_]
                                shift-right: [w662] -> w659
                                shift-left: w660 -> [w662]
                                tunnel: ["0"] -> w656 mode=indexing
                                }
                              }
                              frame True {
                                w668 = TRUE ("Start")
                                n151 = call "WS1021 RFFE Multi Dut Handshake Check.vi"("HS CHK CNTRL"=w675, "TMN DC\\CAP Data Log File Path"=w677, "Debug?"=FALSE, "Set Register"="3", "Select Brd"=enum16{"A", "B"}."B", "Lot#"=w673, "Stop Button"=w668, "Wafer #"=w672, "File Name"=w663, "Error In"=w666, "FPGA"=w671, "SN#"=w670, "Start"=w668) -> ("Status"=w676:string[], "Pass/Fail?"=w664:bool[], "Error Out"=w665:errorcluster)
                              }
                            }
                          }
                        }
                        "Brd A Pass/Fail?" <- w539
                        "Brd B Pass/Fail?" <- w538
                        n152 = call "TLTSP_Measurement.vi"("error in (no error)"=w564, "Select Measurement"=w561, "VISA resource name"=w563) -> ("error out"=w557:errorcluster, "Output"=w553:string, "VISA resource name out"=w562:refnum<visa-resource-name>)  [unwired: 6 in]
                        n153 = call "Time Delay.vi"("Error In"=w557, "Delay(ms)"=u32 100) -> ("Error Out"=w556:errorcluster)  [unwired: 9 in]
                        n154 = call "TLTSP_Measurement.vi"("error in (no error)"=w556, "Select Measurement"=w560, "VISA resource name"=w562) -> ("error out"=w535:errorcluster, "Output"=w554:string, "VISA resource name out"=w558:refnum<visa-resource-name>)  [unwired: 6 in]
                        n155 = case shown="Error" w535 {
                          selector: w535 -> [w592 _]
                          tunnel: [w592 errorcluster {"status"=FALSE, "code"=0, "source"=""} ("error IO")] -> w534
                          tunnel: ["0" "2"] -> w533
                          frame No Error {
                          }
                          frame Error {
                          }
                        }
                        n156 = local write "Temp (C)"(w553) -> ()
                        n157 = for {
                          N: 32 -> [_]
                          shift-right: [w601] -> w575
                          shift-left: w534 -> [w601]
                          tunnel: w574 -> [w600]
                          tunnel: w573 -> [w598]
                          tunnel: w572 -> [w599]
                          tunnel: w571 -> [w597]
                          tunnel: [w600] -> w566 mode=indexing
                          tunnel: [w599] -> w568 mode=indexing
                          tunnel: [w598] -> w567 mode=indexing
                          tunnel: [w597] -> w569 mode=indexing
                          tunnel: [w596] -> w565 mode=indexing
                          tunnel: w553 -> [w596]
                          tunnel: [w595] -> w559 mode=indexing
                          tunnel: w554 -> [w595]
                        }
                        n158 = local write "RH(%)"(w554) -> ()
                        n159 = flat-sequence {
                          tunnel: w575 -> [w701]
                          tunnel: [w701] -> w589
                          tunnel: [w700] -> w590
                          tunnel: w588 -> [w699]
                          tunnel: [w698] -> w587
                          tunnel: w586 -> [w697]
                          tunnel: [w696] -> w585
                          tunnel: w584 -> [w695]
                          tunnel: [w695] -> w583
                          tunnel: w582 -> [w694]
                          tunnel: [w694] -> w581
                          tunnel: w580 -> [w693]
                          tunnel: [w693] -> w579
                          tunnel: w576 -> [w692]
                          tunnel: w545 -> [w691]
                          tunnel: w569 -> [w690]
                          tunnel: w569 -> [w689]
                          tunnel: w568 -> [w683]
                          tunnel: w568 -> [w688]
                          tunnel: w567 -> [w687]
                          tunnel: w567 -> [w686]
                          tunnel: w566 -> [w685]
                          tunnel: w566 -> [w684]
                          tunnel: w565 -> [w682]
                          tunnel: w565 -> [w681]
                          tunnel: w559 -> [w680]
                          tunnel: w559 -> [w679]
                          tunnel: w533 -> [w678]
                          tunnel: [w678] -> w532
                          frame #0 {
                            n160 = Build Array (concatenate)(w699, w691, w690, w683, w687, w685, w682, w680) -> (w698:string[][])
                            n161 = Build Array (concatenate)(w697, w692, w689, w688, w686, w684, w681, w679) -> (w696:string[][])
                            n162 = Select(t=Test_Sequences."Save Data" ("Test Sequences"), s=w701, f=Test_Sequences."Stress" ("Test Sequences")) -> (s? t:f=w700:T8)
                          }
                        }
                      }
                      frame "Stress" {
                        n163 = case shown="False" w751 {
                          tunnel: w750 -> [w783 w981]
                          tunnel: [w785 w978] -> w749
                          tunnel: w748 -> [w784 _]
                          tunnel: w747 -> [w781 _]
                          tunnel: [w780 FALSE ("Abort Stress")] -> w706
                          tunnel: w746 -> [w777 w982]
                          tunnel: w745 -> [_ w980]
                          tunnel: w739 -> [w779 _]
                          tunnel: w738 -> [w775 w977]
                          tunnel: [w774 w977] -> w737
                          tunnel: [w773 u64 1] -> w736
                          tunnel: [w778 "RPM"] -> w734
                          tunnel: w729 -> [w776 _]
                          tunnel: w728 -> [w772 _]
                          tunnel: [w771 "na" ("Cycle DC %")] -> w727
                          tunnel: w726 -> [w770 _]
                          tunnel: w704 -> [w769 _]
                          tunnel: w725 -> [w768 w973]
                          tunnel: [w766 w973] -> w724
                          tunnel: w715 -> [w765 w972]
                          tunnel: [w764 w972] -> w714
                          tunnel: w711 -> [w763 _]
                          tunnel: w712 -> [w762 _]
                          tunnel: w712 -> [w761 _]
                          tunnel: w704 -> [w760 _]
                          tunnel: w710 -> [w759 _]
                          tunnel: w709 -> [w758 _]
                          tunnel: w708 -> [w757 _]
                          tunnel: w704 -> [w754 _]
                          frame False {
                            # "Stress"
                            n164 = case shown="True" w781 {
                              tunnel: w783 -> [w789 w797]
                              tunnel: [w788 w795] -> w782
                              tunnel: w768 -> [w790 w800]
                              tunnel: [w790 w800] -> w767
                              tunnel: w757 -> [w787 w799]
                              tunnel: [w787 w799] -> w756
                              tunnel: [w786 "n/a" ("Beams")] -> w755
                              tunnel: w754 -> [_ w796]
                              frame False {
                                # "Beams"
                                n165 = call "WS1021 Stress Beams.vi"("error in (no error)"=w789, "Cycling Bit"=w787) -> ("error out"=w788:errorcluster, "Beams"=w786:string)  [unwired: 7 in, 1 out]
                              }
                              frame True {
                                # "OTP"
                                n166 = call "WSVCAP SHL Host TL RFFE Write - Multiple DUTs - Common Data.vi"("Data Out"="074100", "error in"=w797, "FPGA"=w796, "Log (T)"=FALSE) -> ("error out"=w793:errorcluster)  [unwired: 11 in]
                                n167 = call "Time Delay.vi"("Error In"=w793, "Delay(ms)"=u32 10) -> ("Error Out"=w795:errorcluster)  [unwired: 9 in]
                              }
                            }
                            n168 = case shown="True" w784 {
                              tunnel: w782 -> [w832 w923]
                              tunnel: [w825 w909] -> w785
                              tunnel: [w836 w926] -> w780
                              tunnel: w779 -> [w830 _]
                              tunnel: [w833 w895] -> w778
                              tunnel: w777 -> [w811 w922]
                              tunnel: w776 -> [w831 w920]
                              tunnel: w775 -> [w822 w925]
                              tunnel: [w819 w924] -> w774
                              tunnel: [w823 w898] -> w773
                              tunnel: w772 -> [_ w921]
                              tunnel: [w818 "Cycle DC %"] -> w771
                              tunnel: w770 -> [w817 w919]
                              tunnel: w769 -> [w812 w905]
                              tunnel: w767 -> [w810 w916]
                              tunnel: [w807 w916] -> w766
                              tunnel: w765 -> [w806 w915]
                              tunnel: [w803 w915] -> w764
                              tunnel: w763 -> [_ w913]
                              tunnel: w762 -> [_ w912]
                              tunnel: w761 -> [_ w908]
                              tunnel: w760 -> [_ w907]
                              tunnel: w759 -> [_ w906]
                              tunnel: w758 -> [_ w896]
                              tunnel: w756 -> [_ w897]
                              tunnel: w755 -> [_ w895]
                              frame False {
                                # "HD"
                                n169 = case shown="15, Default" w811 {
                                tunnel: w832 -> [w838 w840]
                                tunnel: [w838 w840] -> w828
                                tunnel: w831 -> [_ w839]
                                tunnel: [w837 w839] -> w802
                                tunnel: w830 -> [w837 _]
                                frame 15, Default {
                                }
                                frame 0..14 {
                                }
                                }
                                n170 = Format Into String(format string="%s", w817) -> (resulting string=w815:string)  [unwired: 2 in, 1 out]
                                n171 = Concatenate Strings(w815, "_Hold Down..." ("string")) -> (w813:string)
                                n172 = local write "Status"(w813) -> ()
                                n173 = flat-sequence {
                                tunnel: w802 -> [w864]
                                tunnel: [w860] -> w834
                                tunnel: "HD Cmd" -> [w857]
                                tunnel: w828 -> [w858]
                                tunnel: [w845] -> w827
                                tunnel: w822 -> [w859]
                                tunnel: [w859] -> w821
                                tunnel: w812 -> [w846]
                                tunnel: w811 -> [w853]
                                tunnel: w810 -> [w852]
                                tunnel: [w851] -> w809
                                tunnel: w806 -> [w849]
                                tunnel: [w849] -> w805
                                tunnel: w802 -> [w848]
                                tunnel: [w848] -> w801
                                tunnel: [w878] -> w835
                                tunnel: w834 -> [w876]
                                tunnel: w827 -> [w874]
                                tunnel: [w877] -> w826
                                tunnel: [w869] -> w824
                                tunnel: w821 -> [w875]
                                tunnel: [w875] -> w820
                                tunnel: w809 -> [w870]
                                tunnel: [w870] -> w808
                                tunnel: w805 -> [w872]
                                tunnel: [w871] -> w804
                                tunnel: w801 -> [w869]
                                tunnel: [w893] -> w836
                                tunnel: w835 -> [w893]
                                tunnel: ["HD Beams"] -> w833
                                tunnel: w826 -> [w887]
                                tunnel: [w886] -> w825
                                tunnel: w824 -> [w892]
                                tunnel: [w892] -> w823
                                tunnel: w820 -> [w891]
                                tunnel: [w891] -> w819
                                tunnel: ["100"] -> w818
                                tunnel: w808 -> [w888]
                                tunnel: [w888] -> w807
                                tunnel: w804 -> [w885]
                                tunnel: [w884] -> w803
                                frame #0 {
                                n174 = call "WSVCAP SHL Host TL RFFE Write - Multiple DUTs - Common Data.vi"("Data Out"=w857, "error in"=w858, "FPGA"=w846, "Log (T)"=FALSE) -> ("error out"=w855:errorcluster)  [unwired: 11 in]
                                n175 = call "Time Delay.vi"("Error In"=w855, "Delay(ms)"=u32 10) -> ("Error Out"=w850:errorcluster)  [unwired: 9 in]
                                n176 = case shown="1, Default" w853 {
                                tunnel: w852 -> [_ w868]
                                tunnel: [0.0 ("DCV (V)") w868] -> w851
                                tunnel: w850 -> [w866 w867]
                                tunnel: [w866 w867] -> w847
                                frame 0 {
                                }
                                frame 1, Default {
                                }
                                }
                                n177 = Multiply(x=w864, y=u64 1000) -> (x*y=w862:u64)
                                n178 = Multiply(x=w862, y=u64 60) -> (x*y=w860:u64)
                                n179 = call "WS1021 Multi DUT Verify Beam RB.vi"("FPGA"=w846, "Error In"=w847, "Register RB"=string[] ["0762", "0763"]) -> ("Error Out"=w845:errorcluster, "Board B"=w842:string[][], "Board A"=w843:string[][])  [unwired: 6 in]
                                n180 = Build Array (concatenate)(w843, w842) -> (→"RB for HD Stress":string[][])
                                }
                                frame #1 {
                                n181 = call "Ke2400 Configure Output.vi"("error in (no error)"=w874, "Output Level (0)"=w870, "VISA resource name"=w872) -> ("error out"=w873:errorcluster, "VISA resource name out"=w871:refnum<visa-resource-name>)  [unwired: 7 in]
                                n182 = event shown="[0] Timeout" {
                                selector: _ -> [_ _]
                                dyn-events: _ -> [_ _]
                                timeout: w876 -> [_ _]
                                tunnel: ["Abort Stress" TRUE ("Abort Stress")] -> w878
                                tunnel: w873 -> [w880 w882]
                                tunnel: [w880 w882] -> w877
                                event Timeout {
                                n183 = event-data() -> ()  [unwired: 1 in, 2 out]
                                }
                                event "Abort Stress": Value Change {
                                n184 = event-data() -> ()  [unwired: 1 in, 2 out]
                                }
                                }
                                }
                                frame #2 {
                                n185 = call "Ke2400 Configure Output.vi"("error in (no error)"=w887, "Output Level (0)"=0.0, "VISA resource name"=w885) -> ("error out"=w886:errorcluster, "VISA resource name out"=w884:refnum<visa-resource-name>)  [unwired: 7 in]
                                }
                                }
                              }
                              frame True {
                                # "Cycling"
                                n186 = Format Into String(format string="%s", w919) -> (resulting string=w917:string)  [unwired: 2 in, 1 out]
                                n187 = case shown="8, Default" w922 {
                                tunnel: w923 -> [w928 w930]
                                tunnel: [w928 w930] -> w914
                                tunnel: w921 -> [_ w929]
                                tunnel: [w927 w929] -> w900
                                tunnel: w920 -> [w927 _]
                                frame 0..7 {
                                }
                                frame 8, Default {
                                }
                                }
                                n188 = Array Max & Min(array=w896) -> (max value=w904:dbl)  [unwired: 3 out]
                                n189 = call "WSVCAP SHL Host TL RFFE Configure.vi"("RFFE Slave Address"=w912, "Clock Rate (Hz)"=w913, "error in"=w914, "FPGA"=w905) -> ("error out"=w911:errorcluster)  [unwired: 10 in, 1 out]
                                n190 = Multiply(x=w900, y=u64 1000) -> (x*y=w898:u64)
                                n191 = Divide(x=1.0, y=w904) -> (x/y=w902:dbl)
                                n192 = To Unsigned Quad Integer(1:w902) -> (0:w901:u64)
                                n193 = while {
                                tunnel: w911 -> [w945]
                                tunnel: [w951] -> w926
                                tunnel: [w935] -> w910
                                tunnel: w925 -> [w950]
                                tunnel: [w950] -> w924
                                tunnel: w917 -> [w948]
                                tunnel: w897 -> [w944]
                                tunnel: w896 -> [w943]
                                tunnel: w905 -> [w931]
                                tunnel: w901 -> [w938]
                                tunnel: w898 -> [w940]
                                i -> [w946]
                                stop <- w952 stop-if-true
                                n194 = case shown="0" w946 {
                                tunnel: w945 -> [w968 w970]
                                tunnel: w944 -> [w965 _]
                                tunnel: w943 -> [w964 _]
                                tunnel: w931 -> [w967 _]
                                tunnel: [w969 w970] -> w934
                                frame 0 {
                                n195 = call "WSVCAP SHL Host TL RFFE Write Cycle - Multiple DUTs - Common Data.vi"("Data Out (Cycle Commands)"=w965, "Post Command Delay"=w964, "error in"=w968, "FPGA"=w967, "Log (T)"=FALSE) -> ("error out"=w969:errorcluster)  [unwired: 10 in]
                                }
                                frame 1, Default {
                                }
                                }
                                n196 = call "WSVCAP SHL Host TL SPI_RFFE Query Cycle Count.vi"("error in"=w934, "FPGA"=w931) -> ("Cycle Count"=w932:u64, "error out"=w933:errorcluster)  [unwired: 12 in]
                                "Cycle Count" <- w932
                                n197 = Concatenate Strings(w948, "_Cycling..." ("string")) -> (w949:string)
                                n198 = local write "Status"(w949) -> ()
                                n199 = Greater Or Equal?(x=w932, y=w940) -> (x >= y?=w942:bool)
                                n200 = Subtract(x=w940, y=w932) -> (x-y=w939:u64)
                                n201 = case shown="True" w942 {
                                tunnel: w933 -> [w957 w961]
                                tunnel: w931 -> [_ w960]
                                tunnel: [FALSE TRUE] -> w941
                                tunnel: [w957 w962] -> w936
                                frame False {
                                }
                                frame True {
                                n202 = call "WSVCAP SHL Host TL RFFE Stop Write Cycle.vi"("error in"=w961, "FPGA"=w960, "Log (T)"=FALSE) -> ("error out"=w962:errorcluster)  [unwired: 12 in]
                                }
                                }
                                n203 = Greater?(x=w939, y=w938) -> (0:w937:bool)
                                n204 = local read "Abort Stress"() -> (w951:bool)
                                n205 = case shown="True" w937 {
                                tunnel: w936 -> [w953 w956]
                                tunnel: [w953 w955] -> w935
                                frame False {
                                }
                                frame True {
                                n206 = call "MISC Wait with Data Flow.vi"("Error In (no error)"=w956, "Wait Time (500ms)"=u32 50) -> ("Error Out"=w955:errorcluster)  [unwired: 7 in, 2 out]
                                }
                                }
                                n207 = Or(x=w951, y=w941) -> (x .or. y?=w952:bool)
                                }
                                n208 = call "WSVCAP SHL Host TL RFFE Configure.vi"("RFFE Slave Address"=w908, "Clock Rate (Hz)"=w906, "error in"=w910, "FPGA"=w907) -> ("error out"=w909:errorcluster)  [unwired: 10 in, 1 out]
                                "Verify Bits to Cycle" <- w897
                                "Verify DC Speed" <- w896
                              }
                            }
                          }
                          frame True {
                            # "Verify Socket"
                            n209 = To Unsigned Long Integer(number=w980) -> (unsigned 32bit integer=w979:u32)
                            n210 = case shown="1, Default" w982 {
                              tunnel: w981 -> [w984 w989]
                              tunnel: [w984 w988] -> w978
                              tunnel: w979 -> [_ w987]
                              frame 0 {
                              }
                              frame 1, Default {
                                n211 = Multiply(x=w987, y=u32 1000) -> (x*y=w986:u32)
                                n212 = call "Time Delay.vi"("Error In"=w989, "Delay(ms)"=w986) -> ("Error Out"=w988:errorcluster)  [unwired: 9 in]
                              }
                            }
                            n213 = local write "Status"("RPM to Verify Socket..." ("Status")) -> ()
                          }
                        }
                        n214 = flat-sequence {
                          tunnel: w749 -> [w1004]
                          tunnel: [w1003] -> w752
                          tunnel: [Test_Sequences."I_Measure" ("Test Sequences")] -> w753
                          tunnel: w741 -> [w999]
                          tunnel: w740 -> [w997]
                          tunnel: w737 -> [w1006]
                          tunnel: w736 -> [w1005]
                          tunnel: [w998] -> w735
                          tunnel: w734 -> [w1000]
                          tunnel: [w999] -> w733
                          tunnel: [w996] -> w717
                          tunnel: [w995] -> w719
                          tunnel: [w997] -> w730
                          tunnel: [w996] -> w721
                          tunnel: [w995] -> w723
                          tunnel: w727 -> [w994]
                          tunnel: [w993] -> w722
                          tunnel: [w993] -> w718
                          tunnel: w724 -> [w992]
                          tunnel: [w991] -> w720
                          tunnel: [w991] -> w716
                          tunnel: w714 -> [w990]
                          tunnel: [w990] -> w713
                          frame #0 {
                            n215 = Add(x=w1006, y=w1005) -> (x+y=w998:u64)
                            "TTF Completed" <- w998
                            n216 = for {
                              N: 32 -> [_]
                              shift-right: [w1015] -> w1003
                              shift-left: w1004 -> [w1015]
                              tunnel: w998 -> [w1014]
                              tunnel: [w1012] -> w995 mode=indexing
                              tunnel: w1000 -> [w1011]
                              tunnel: [w1011] -> w996 mode=indexing
                              tunnel: [w1010] -> w993 mode=indexing
                              tunnel: w994 -> [w1010]
                              tunnel: w992 -> [w1009]
                              tunnel: [w1008] -> w991 mode=indexing
                              n217 = Number To Fractional String(number=w1009, precision (6)=i16 2) -> (F-format string=w1008:string)  [unwired: 2 in]
                              n218 = Number To Fractional String(number=w1014, precision (6)=i16 2) -> (F-format string=w1012:string)  [unwired: 2 in]
                            }
                            "Stress DC(%)" <- w994
                          }
                        }
                        n219 = Build Array (concatenate)(w733, w716, w717, w718, w719) -> (w732:string[][])
                        n220 = Build Array (concatenate)(w730, w720, w721, w722, w723) -> (w731:string[][])
                      }
                      frame "I_Measure" {
                        w1029 = FALSE ("true")
                        n221 = stacked-sequence {
                          seq-local: [w1080 _ _] -> [_ w1092 _]
                          seq-local: [w1073 _ _] -> [_ w1088 _]
                          seq-local: [_ w1090 _] -> [_ _ w1111]
                          seq-local: [_ w1089 _] -> [_ _ w1114]
                          tunnel: w1046 -> [w1078 _ _]
                          tunnel: u32 100 ("Delay(ms)") -> [w1083 w1085 w1115]
                          tunnel: w1044 -> [w1081 _ _]
                          tunnel: [w1079 _ _] -> w1036
                          tunnel: [_ w1091 _] -> w1035
                          tunnel: [_ _ w1113] -> w1043
                          tunnel: [_ _ w1106] -> w1032
                          tunnel: [_ _ w1112] -> w1034
                          tunnel: w1037 -> [w1075 w1087 w1105]
                          tunnel: [_ _ w1101] -> w1024
                          tunnel: [_ _ w1100] -> w1022
                          frame #0 {
                            # "IDD Stdby"
                            n222 = call "WSVCAP SHL Host TL RFFE Write - Multiple DUTs - Common Data.vi"("Data Out"="074000", "error in"=w1078, "FPGA"=w1075, "Log (T)"=FALSE) -> ("error out"=w1077:errorcluster)  [unwired: 11 in]
                            n223 = call "Time Delay.vi"("Error In"=w1077, "Delay(ms)"=w1083) -> ("Error Out"=w1082:errorcluster)  [unwired: 9 in]
                            n224 = call "Ke2000 Single Reading.vi"("error in (no error)"=w1082, "VISA resource name"=w1081) -> ("error out"=w1073:errorcluster, "VISA resource name out"=w1080:refnum<visa-resource-name>, "uA"=w1079:string)  [unwired: 5 in, 2 out]
                          }
                          frame #1 {
                            # "IDD ALL ON"
                            n225 = for {
                              tunnel: w1087 -> [w1097]
                              shift-right: [w1094] -> w1084
                              shift-left: w1088 -> [w1098]
                              tunnel: string[] ["074080", "074101", "0701027F7F"] -> [w1096] mode=indexing
                              tunnel: w1085 -> [w1093]
                              n226 = call "WSVCAP SHL Host TL RFFE Write - Multiple DUTs - Common Data.vi"("Data Out"=w1096, "error in"=w1098, "FPGA"=w1097, "Log (T)"=FALSE) -> ("error out"=w1095:errorcluster)  [unwired: 11 in]
                              n227 = call "Time Delay.vi"("Error In"=w1095, "Delay(ms)"=w1093) -> ("Error Out"=w1094:errorcluster)  [unwired: 9 in]
                            }
                            n228 = call "Ke2000 Single Reading.vi"("error in (no error)"=w1084, "VISA resource name"=w1092) -> ("error out"=w1090:errorcluster, "VISA resource name out"=w1089:refnum<visa-resource-name>, "uA"=w1091:string)  [unwired: 5 in, 2 out]
                          }
                          frame #2 {
                            # "IDD ALL OFF"
                            n229 = call "WSVCAP SHL Host TL RFFE Write - Multiple DUTs - Common Data.vi"("Data Out"="0701020000", "error in"=w1111, "FPGA"=w1105, "Log (T)"=FALSE) -> ("error out"=w1110:errorcluster)  [unwired: 11 in]
                            n230 = call "Time Delay.vi"("Error In"=w1110, "Delay(ms)"=w1115) -> ("Error Out"=w1116:errorcluster)  [unwired: 9 in]
                            n231 = call "Ke2000 Single Reading.vi"("error in (no error)"=w1116, "VISA resource name"=w1114) -> ("error out"=w1107:errorcluster, "VISA resource name out"=w1113:refnum<visa-resource-name>, "uA"=w1112:string)  [unwired: 5 in, 2 out]
                            n232 = call "WS1021 ADI Read 64 DUT.vi"("FPGA"=w1105, "Error In"=w1107) -> ("Error Out"=w1106:errorcluster, "AD7747 Values"=w1103:string[][])  [unwired: 8 in]
                            n233 = Index Array(array=w1103, index (col)=5 ("disabled index (col)")) -> (element=w1101:string[])  [unwired: 1 in]
                            n234 = Index Array(array=w1103, index (col)=2 ("disabled index (col)")) -> (element=w1100:string[])  [unwired: 1 in]
                          }
                        }
                        n235 = local write "Status"("Measure IDD..." ("Status")) -> ()
                        n236 = Build Array(w1036, w1035, w1034) -> (→"IDD Measurement(uA)":string[])
                        n237 = for {
                          N: 32 -> [_]
                          tunnel: w1036 -> [w1072]
                          tunnel: [w1072] -> w1041 mode=indexing
                          tunnel: w1035 -> [w1071]
                          tunnel: [w1071] -> w1040 mode=indexing
                          tunnel: w1034 -> [w1070]
                          tunnel: [w1070] -> w1039 mode=indexing
                          shift-right: [w1069] -> w1021
                          shift-left: w1032 -> [w1069]
                        }
                        n238 = case shown="True" w1025 {
                          tunnel: w1024 -> [_ w1064]
                          tunnel: [string[] [] ("AD7747 Values") w1064] -> w1016
                          tunnel: w1021 -> [w1061 w1063]
                          tunnel: [w1061 w1063] -> w1019
                          frame False {
                          }
                          frame True {
                          }
                        }
                        "Cmin BrdB" <- w1016
                        n239 = case shown="True" w1023 {
                          tunnel: w1022 -> [_ w1060]
                          tunnel: [string[] [] ("AD7747 Values") w1060] -> w1017
                          tunnel: w1021 -> [w1058 w1059]
                          tunnel: [w1058 w1059] -> w1018
                          frame False {
                          }
                          frame True {
                          }
                        }
                        "Cmin BrdA" <- w1017
                        n240 = Fract/Exp String To Number(string=w1017) -> (number=→"CMin BrdA (fF)":dbl[])  [unwired: 3 in, 1 out]
                        n241 = Fract/Exp String To Number(string=w1016) -> (number=→"CMin BrdB (fF)":dbl[])  [unwired: 3 in, 1 out]
                        n242 = Merge Errors(w1019, w1018) -> (w1020:errorcluster)
                        n243 = case shown="Error" w1020 {
                          selector: w1020 -> [w1065 _]
                          tunnel: ["0" "3"] -> w1026
                          tunnel: [w1065 errorcluster {"status"=FALSE, "code"=0, "source"=""} ("Error Out")] -> w1027
                          frame No Error {
                          }
                          frame Error {
                          }
                        }
                        n244 = flat-sequence {
                          tunnel: w1027 -> [w1131]
                          tunnel: [w1131] -> w1055
                          tunnel: [w1130] -> w1056
                          tunnel: w1053 -> [w1129]
                          tunnel: [w1128] -> w1052
                          tunnel: [w1127] -> w1051
                          tunnel: w1050 -> [w1126]
                          tunnel: w1041 -> [w1125]
                          tunnel: w1041 -> [w1124]
                          tunnel: w1040 -> [w1123]
                          tunnel: w1040 -> [w1122]
                          tunnel: w1039 -> [w1121]
                          tunnel: w1039 -> [w1120]
                          tunnel: w1024 -> [w1118]
                          tunnel: w1022 -> [w1119]
                          tunnel: w1026 -> [w1117]
                          tunnel: [w1117] -> w1028
                          frame #0 {
                            n245 = Build Array (concatenate)(w1129, w1125, w1123, w1121, w1118) -> (w1128:string[][])
                            n246 = Build Array (concatenate)(w1126, w1124, w1122, w1120, w1119) -> (w1127:string[][])
                            n247 = Select(t=Test_Sequences."Save Data" ("Test Sequences"), s=w1131, f=Test_Sequences."Cap_Measure" ("Test Sequences")) -> (s? t:f=w1130:T8)
                          }
                        }
                      }
                      frame "Cap_Measure" {
                        w1137 = FALSE ("true")
                        n248 = Build Array (concatenate)(w1170, w1169) -> (w1168:string[])
                        n249 = Build Array (concatenate)(w1173, w1172) -> (w1171:string[])
                        n250 = call "WS1021 CP Setting.vi"("Manual Setting"=w1139, "FPGA"=w1140, "Error In"=w1144) -> ("Error Out"=w1142:errorcluster)  [unwired: 7 in, 1 out]
                        n251 = call "Time Delay.vi"("Error In"=w1142, "Delay(ms)"=u32 50) -> ("Error Out"=w1143:errorcluster)  [unwired: 9 in]
                        n252 = for {
                          shift-right: [w1212] -> w1163
                          shift-left: w1143 -> [w1223]
                          tunnel: w1171 -> [w1222] mode=indexing
                          tunnel: w1168 -> [w1227] mode=indexing
                          tunnel: [w1215] -> w1159 mode=indexing
                          tunnel: [w1224] -> w1161 mode=indexing
                          tunnel: w1138 -> [w1221]
                          tunnel: w1138 -> [w1214]
                          n253 = call "WSVCAP SHL Host TL RFFE Write - Multiple DUTs - Common Data.vi"("Data Out"=w1222, "error in"=w1223, "FPGA"=w1221, "Log (T)"=FALSE) -> ("error out"=w1219:errorcluster)  [unwired: 11 in]
                          n254 = Concatenate Strings("Measure " ("string"), w1227) -> (w1225:string)
                          n255 = local write "Status"(w1225) -> ()
                          n256 = call "WS1021 ADI Read 64 DUT.vi"("FPGA"=w1214, "Error In"=w1219) -> ("Error Out"=w1213:errorcluster, "AD7747 Values"=w1216:string[][])  [unwired: 8 in]
                          n257 = Index Array(array=w1216, index (col)=5 ("disabled index (col)")) -> (element=w1224:string[])  [unwired: 1 in]
                          n258 = Index Array(array=w1216, index (col)=2 ("disabled index (col)")) -> (element=w1215:string[])  [unwired: 1 in]
                          n259 = call "Time Delay.vi"("Error In"=w1213, "Delay(ms)"=u32 10) -> ("Error Out"=w1212:errorcluster)  [unwired: 9 in]
                        }
                        n260 = case shown="True" w1135 {
                          tunnel: w1163 -> [w1193 w1202]
                          tunnel: w1161 -> [_ w1201]
                          tunnel: [string[][] [] w1200] -> w1160
                          tunnel: [_ w1199] -> w1157
                          tunnel: [_ w1198] -> w1155
                          tunnel: [_ w1197] -> w1153
                          tunnel: [_ w1196] -> w1151
                          tunnel: [w1193 w1195] -> w1148
                          frame False {
                          }
                          frame True {
                            n261 = Transpose 2D Array(2D array=w1201) -> (transposed array=w1200:string[][])
                            n262 = local read "CMin BrdB (fF)"() -> (w1194:dbl[])
                            n263 = call "WS1021 Calc DCAP_RTZ_Percentage.vi"("Cmin(fF)"=w1194, "Error In"=w1202, "Input"=w1200) -> ("Error Out"=w1195:errorcluster, "% Total Delta C(fF)"=w1197:string[], "Total Delta C(fF)"=w1198:string[], "% Beam Delta C(fF)"=w1199:string[][], "Delta Cap(fF)"=w1196:string[][])  [unwired: 3 in, 1 out]
                          }
                        }
                        "Brd B_Beam Cap (fF)" <- w1160
                        n264 = case shown="True" w1134 {
                          tunnel: w1163 -> [w1182 w1191]
                          tunnel: w1159 -> [_ w1190]
                          tunnel: [string[][] [] w1189] -> w1158
                          tunnel: [_ w1188] -> w1156
                          tunnel: [_ w1187] -> w1154
                          tunnel: [_ w1186] -> w1152
                          tunnel: [_ w1185] -> w1150
                          tunnel: [w1182 w1184] -> w1146
                          frame False {
                          }
                          frame True {
                            n265 = Transpose 2D Array(2D array=w1190) -> (transposed array=w1189:string[][])
                            n266 = local read "CMin BrdA (fF)"() -> (w1183:dbl[])
                            n267 = call "WS1021 Calc DCAP_RTZ_Percentage.vi"("Cmin(fF)"=w1183, "Error In"=w1191, "Input"=w1189) -> ("Error Out"=w1184:errorcluster, "% Total Delta C(fF)"=w1186:string[], "Total Delta C(fF)"=w1187:string[], "% Beam Delta C(fF)"=w1188:string[][], "Delta Cap(fF)"=w1185:string[][])  [unwired: 3 in, 1 out]
                          }
                        }
                        "Brd A_Beam Cap (fF)" <- w1158
                        n268 = case shown="1, Default" w1149 {
                          tunnel: w1153 -> [w1206 w1208]
                          tunnel: w1152 -> [w1205 w1207]
                          tunnel: w1148 -> [w1204 w1210]
                          tunnel: [w1204 w1210] -> w1147
                          tunnel: w1146 -> [w1203 w1209]
                          tunnel: [w1203 w1209] -> w1145
                          frame 0 {
                            "T0_Brd A Delta C%" <- w1205
                            "T0_Brd B Delta C%" <- w1206
                          }
                          frame 1, Default {
                            "Brd B Delta C%" <- w1208
                            "Brd A Delta C%" <- w1207
                          }
                        }
                        n269 = Merge Errors(w1147, w1145) -> (w1162:errorcluster)
                        n270 = flat-sequence {
                          tunnel: w1162 -> [w1244]
                          tunnel: [w1244] -> w1179
                          tunnel: [w1243] -> w1180
                          tunnel: w1167 -> [w1239]
                          tunnel: [w1242] -> w1166
                          tunnel: w1165 -> [w1236]
                          tunnel: [w1241] -> w1164
                          tunnel: w1159 -> [w1235]
                          tunnel: w1161 -> [w1238]
                          tunnel: w1157 -> [w1240]
                          tunnel: w1156 -> [w1233]
                          tunnel: w1155 -> [w1232]
                          tunnel: w1154 -> [w1230]
                          tunnel: w1153 -> [w1231]
                          tunnel: w1152 -> [w1229]
                          tunnel: w1151 -> [w1237]
                          tunnel: w1150 -> [w1234]
                          tunnel: [""] -> w1136
                          frame #0 {
                            n271 = Build Array (concatenate)(w1239, w1238, w1237, w1240, w1232, w1231) -> (w1242:string[][])
                            n272 = Build Array (concatenate)(w1236, w1235, w1234, w1233, w1230, w1229) -> (w1241:string[][])
                            n273 = Select(t=Test_Sequences."Save Data" ("Test Sequences"), s=w1244, f=Test_Sequences."VPI" ("Test Sequences")) -> (s? t:f=w1243:T8)
                          }
                        }
                      }
                      frame "VPI" {
                        w1255 = FALSE ("true")
                        n274 = case shown="True" w1275 {
                          tunnel: w1279 -> [w1311 w1338]
                          tunnel: w1278 -> [w1314 w1341]
                          tunnel: w1277 -> [_ w1340]
                          tunnel: [w1315 w1339] -> w1267
                          tunnel: w1270 -> [_ w1337]
                          tunnel: w1269 -> [_ w1336]
                          tunnel: w1268 -> [_ w1333]
                          tunnel: [w1313 w1332] -> w1254
                          tunnel: [w1312 w1331] -> w1253
                          tunnel: [w1308 w1327] -> w1249
                          frame False {
                            n275 = for {
                              N: 32 -> [_]
                              shift-right: [w1317] -> w1310
                              shift-left: w1311 -> [w1317]
                              tunnel: [""] -> w1308 mode=indexing
                            }
                            n276 = for {
                              tunnel: w1314 -> [w1321] mode=indexing
                              tunnel: [w1320] -> w1313 mode=indexing
                              shift-right: [w1322] -> w1315
                              shift-left: w1310 -> [w1323]
                              tunnel: [w1318] -> w1312 mode=indexing
                              n277 = for {
                                N: 32 -> [_]
                                shift-right: [w1325] -> w1322
                                shift-left: w1323 -> [w1325]
                                tunnel: w1321 -> [_]
                                tunnel: [w1324] -> w1320 mode=indexing
                                tunnel: [w1324] -> w1318 mode=indexing
                                w1324 = ""
                              }
                            }
                          }
                          frame True {
                            n278 = call "WS1021 CP Setting.vi"("Manual Setting"=w1336, "FPGA"=w1337, "Error In"=w1338) -> ("Error Out"=w1330:errorcluster, "CP Select"=w1328:string)  [unwired: 7 in]
                            n279 = for {
                              N: 32 -> [_]
                              shift-right: [w1343] -> w1329
                              shift-left: w1330 -> [w1343]
                              tunnel: w1328 -> [w1342]
                              tunnel: [w1342] -> w1327 mode=indexing
                            }
                            n280 = call "Time Delay.vi"("Error In"=w1329, "Delay(ms)"=u32 50) -> ("Error Out"=w1334:errorcluster)  [unwired: 9 in]
                            n281 = for {
                              shift-right: [w1346] -> w1339
                              shift-left: w1334 -> [w1354]
                              tunnel: w1341 -> [w1359] mode=indexing
                              tunnel: w1340 -> [w1352] mode=indexing
                              tunnel: w1333 -> [w1353]
                              tunnel: [w1348] -> w1332 mode=indexing
                              tunnel: [w1347] -> w1331 mode=indexing
                              n282 = call "WSVCAP SHL Host TL RFFE Write - Multiple DUTs - Common Data.vi"("Data Out"=w1352, "error in"=w1354, "FPGA"=w1353, "Log (T)"=FALSE) -> ("error out"=w1356:errorcluster)  [unwired: 11 in]
                              n283 = call "WS1021 ADI Read 64 DUT.vi"("FPGA"=w1353, "Error In"=w1356) -> ("Error Out"=w1345:errorcluster, "AD7747 Values"=w1351:string[][])  [unwired: 8 in]
                              n284 = Concatenate Strings("Measure VPI " ("string"), w1359) -> (w1357:string)
                              n285 = local write "Status"(w1357) -> ()
                              n286 = Index Array(array=w1351, index (col)=5 ("disabled index (col)")) -> (element=w1348:string[])  [unwired: 1 in]
                              n287 = Index Array(array=w1351, index (col)=2 ("disabled index (col)")) -> (element=w1347:string[])  [unwired: 1 in]
                              n288 = call "Time Delay.vi"("Error In"=w1345, "Delay(ms)"=u32 10) -> ("Error Out"=w1346:errorcluster)  [unwired: 9 in]
                            }
                          }
                        }
                        n289 = case shown="True" w1247 {
                          tunnel: w1267 -> [w1299 w1307]
                          tunnel: [w1299 w1306] -> w1265
                          tunnel: [_ w1305] -> w1263
                          tunnel: [_ w1304] -> w1262
                          tunnel: [_ w1303] -> w1261
                          tunnel: [string[] [] ("VPI % Delta C") w1302] -> w1260
                          tunnel: w1254 -> [_ w1301]
                          tunnel: [string[][] [] w1300] -> w1251
                          frame False {
                          }
                          frame True {
                            n290 = Transpose 2D Array(2D array=w1301) -> (transposed array=w1300:string[][])
                            n291 = call "WS1021 Multi DUT VPI DeltaC.vi"("Error In"=w1307, "VPI Input"=w1300) -> ("Error Out"=w1306:errorcluster, "VPI % Delta C"=w1302:string[], "VPI Total Delta C (fF)"=w1303:string[], "VPI Delta C R2 (fF)"=w1304:string[], "VPI Delta C R3 (fF)"=w1305:string[])  [unwired: 5 in]
                          }
                        }
                        "VPI Brd B Delta C%" <- w1260
                        "Brd B_VPI Cap (fF)" <- w1251
                        n292 = case shown="True" w1248 {
                          tunnel: w1267 -> [w1288 w1296]
                          tunnel: [w1288 w1295] -> w1264
                          tunnel: [_ w1294] -> w1259
                          tunnel: [_ w1293] -> w1258
                          tunnel: [_ w1292] -> w1257
                          tunnel: [string[] [] ("VPI % Delta C") w1291] -> w1256
                          tunnel: w1253 -> [_ w1290]
                          tunnel: [string[][] [] w1289] -> w1252
                          frame False {
                          }
                          frame True {
                            n293 = Transpose 2D Array(2D array=w1290) -> (transposed array=w1289:string[][])
                            n294 = call "WS1021 Multi DUT VPI DeltaC.vi"("Error In"=w1296, "VPI Input"=w1289) -> ("Error Out"=w1295:errorcluster, "VPI % Delta C"=w1291:string[], "VPI Total Delta C (fF)"=w1292:string[], "VPI Delta C R2 (fF)"=w1293:string[], "VPI Delta C R3 (fF)"=w1294:string[])  [unwired: 5 in]
                          }
                        }
                        "VPI Brd A Delta C%" <- w1256
                        "Brd A_VPI Cap (fF)" <- w1252
                        n295 = Merge Errors(w1265, w1264) -> (w1266:errorcluster)
                        n296 = flat-sequence {
                          tunnel: w1266 -> [w1378]
                          tunnel: [w1378] -> w1285
                          tunnel: [w1377] -> w1284
                          tunnel: [w1376] -> w1274
                          tunnel: w1273 -> [w1375]
                          tunnel: w1272 -> [w1374]
                          tunnel: [w1373] -> w1271
                          tunnel: w1254 -> [w1367]
                          tunnel: w1253 -> [w1361]
                          tunnel: w1263 -> [w1368]
                          tunnel: w1262 -> [w1369]
                          tunnel: w1261 -> [w1370]
                          tunnel: w1260 -> [w1371]
                          tunnel: w1259 -> [w1363]
                          tunnel: w1258 -> [w1364]
                          tunnel: w1257 -> [w1365]
                          tunnel: w1256 -> [w1366]
                          tunnel: [""] -> w1250
                          tunnel: w1249 -> [w1362]
                          tunnel: w1249 -> [w1360]
                          frame #0 {
                            n297 = Build Array (concatenate)(w1375, w1362, w1367, w1368, w1369, w1370, w1371) -> (w1376:string[][])
                            n298 = Build Array (concatenate)(w1374, w1360, w1361, w1363, w1364, w1365, w1366) -> (w1373:string[][])
                            n299 = Select(t=Test_Sequences."Save Data" ("Test Sequences"), s=w1378, f=Test_Sequences."Open State VCmin" ("Test Sequences")) -> (s? t:f=w1377:T8)
                          }
                        }
                      }
                      frame "Open State VCmin" {
                        w1389 = FALSE ("true")
                        n300 = case shown="False" w1418 {
                          tunnel: w1417 -> [w1459 w1480]
                          tunnel: w1416 -> [w1455 w1479]
                          tunnel: w1415 -> [w1457 w1478]
                          tunnel: [w1458 w1477] -> w1407
                          tunnel: [w1456 w1476] -> w1393
                          tunnel: [w1455 w1475] -> w1410
                          tunnel: [w1454 w1474] -> w1392
                          tunnel: [w1453 w1473] -> w1391
                          tunnel: w1390 -> [_ w1472]
                          frame False {
                            n301 = for {
                              shift-right: [w1465] -> w1458
                              shift-left: w1459 -> [w1466]
                              tunnel: w1457 -> [w1468] mode=indexing
                              tunnel: [w1462] -> w1456 mode=indexing
                              tunnel: [w1461] -> w1454 mode=indexing
                              tunnel: [w1460] -> w1453 mode=indexing
                              n302 = Number To Fractional String(number=w1468, precision (6)=i16 2) -> (F-format string=w1463:string)  [unwired: 2 in]
                              n303 = for {
                                N: 32 -> [_]
                                shift-right: [w1471] -> w1465
                                shift-left: w1466 -> [w1471]
                                tunnel: w1463 -> [w1470]
                                tunnel: [w1470] -> w1462 mode=indexing
                                tunnel: [w1469] -> w1461 mode=indexing
                                tunnel: [w1469] -> w1460 mode=indexing
                                w1469 = ""
                              }
                            }
                          }
                          frame True {
                            n304 = for {
                              tunnel: w1479 -> [w1506]
                              tunnel: w1478 -> [w1504] mode=indexing
                              tunnel: [w1492] -> w1476 mode=indexing
                              shift-right: [w1488] -> w1477
                              shift-left: w1480 -> [w1507]
                              tunnel: [w1491] -> w1475
                              tunnel: [w1485] -> w1474 mode=indexing
                              tunnel: [w1484] -> w1473 mode=indexing
                              tunnel: w1472 -> [w1481]
                              n305 = call "Ke2400 Configure Output.vi"("error in (no error)"=w1507, "Compliance  Level (0.1)"=0.1, "Output Level (0)"=w1504, "VISA resource name"=w1506) -> ("error out"=w1500:errorcluster, "VISA resource name out"=w1499:refnum<visa-resource-name>)  [unwired: 6 in]
                              n306 = Number To Fractional String(number=w1504, precision (6)=i16 2) -> (F-format string=w1494:string)  [unwired: 2 in]
                              n307 = Concatenate Strings("Testing OS " ("string"), w1494) -> (w1501:string)
                              n308 = call "Ke2400 Enable.vi"("error in (no error)"=w1500, "ON/OFF"=TRUE, "VISA In"=w1499) -> ("error out"=w1497:errorcluster, "VISA Out"=w1491:refnum<visa-resource-name>)  [unwired: 7 in]
                              n309 = call "Time Delay.vi"("Error In"=w1497, "Delay(ms)"=u32 10) -> ("Error Out"=w1495:errorcluster)  [unwired: 9 in]
                              n310 = for {
                                N: 32 -> [_]
                                shift-right: [w1509] -> w1490
                                shift-left: w1495 -> [w1509]
                                tunnel: w1494 -> [w1508]
                                tunnel: [w1508] -> w1492 mode=indexing
                              }
                              n311 = local write "Status"(w1501) -> ()
                              n312 = call "WS1021 ADI Read 64 DUT.vi"("FPGA"=w1481, "Error In"=w1490) -> ("Error Out"=w1489:errorcluster, "AD7747 Values"=w1486:string[][])  [unwired: 8 in]
                              n313 = Index Array(array=w1486, index (col)=5 ("disabled index (col)")) -> (element=w1485:string[])  [unwired: 1 in]
                              n314 = Index Array(array=w1486, index (col)=2 ("disabled index (col)")) -> (element=w1484:string[])  [unwired: 1 in]
                              n315 = call "Time Delay.vi"("Error In"=w1489, "Delay(ms)"=u32 50) -> ("Error Out"=w1488:errorcluster)  [unwired: 9 in]
                            }
                          }
                        }
                        n316 = case shown="True" w1382 {
                          tunnel: w1407 -> [w1438 w1448]
                          tunnel: [w1438 w1447] -> w1405
                          tunnel: [_ w1446] -> w1403
                          tunnel: [_ w1445] -> w1402
                          tunnel: [_ w1444] -> w1401
                          tunnel: [w1437 w1443] -> w1396
                          tunnel: [w1437 w1442] -> w1395
                          tunnel: [w1437 w1441] -> w1394
                          tunnel: w1393 -> [_ w1440]
                          tunnel: w1392 -> [_ w1439]
                          frame False {
                            w1437 = string[][] [] ("VSA_V3")
                          }
                          frame True {
                            n317 = call "WS1021 VSA Convert Data.vi"("VSA_Cap(fF)"=w1439, "Voltage(V)"=w1440, "error in (no error)"=w1448) -> ("BT_VSA_V1"=w1446:string[][], "BT_VSA_V2"=w1445:string[][], "BT_VSA_V3"=w1444:string[][], "VSA_V3"=w1443:string[][], "VSA_V1"=w1441:string[][], "VSA_V2"=w1442:string[][], "error out"=w1447:errorcluster)  [unwired: 6 in]
                          }
                        }
                        "Brd B_OS_V1 (fF)" <- w1394
                        "Brd B_OS_V2 (fF)" <- w1395
                        "Brd B_OS_V3 (fF)" <- w1396
                        n318 = case shown="True" w1381 {
                          tunnel: w1407 -> [w1426 w1436]
                          tunnel: [w1426 w1435] -> w1404
                          tunnel: [_ w1434] -> w1400
                          tunnel: [_ w1433] -> w1399
                          tunnel: [_ w1432] -> w1398
                          tunnel: [w1425 w1431] -> w1397
                          tunnel: w1393 -> [_ w1430]
                          tunnel: w1391 -> [_ w1429]
                          tunnel: [w1425 w1428] -> w1388
                          tunnel: [w1425 w1427] -> w1387
                          frame False {
                            w1425 = string[][] [] ("VSA_V3")
                          }
                          frame True {
                            n319 = call "WS1021 VSA Convert Data.vi"("VSA_Cap(fF)"=w1429, "Voltage(V)"=w1430, "error in (no error)"=w1436) -> ("BT_VSA_V1"=w1434:string[][], "BT_VSA_V2"=w1433:string[][], "BT_VSA_V3"=w1432:string[][], "VSA_V3"=w1431:string[][], "VSA_V1"=w1428:string[][], "VSA_V2"=w1427:string[][], "error out"=w1435:errorcluster)  [unwired: 6 in]
                          }
                        }
                        "Brd A_OS_V2 (fF)" <- w1387
                        "Brd A_OS_V3 (fF)" <- w1397
                        "Brd A_OS_V1 (fF)" <- w1388
                        n320 = Merge Errors(w1405, w1404) -> (w1406:errorcluster)
                        n321 = call "Ke2400 Configure Output.vi"("error in (no error)"=w1406, "Output Level (0)"=0.0, "VISA resource name"=w1410) -> ("error out"=w1386:errorcluster, "VISA resource name out"=w1409:refnum<visa-resource-name>)  [unwired: 7 in]
                        n322 = case shown="Error" w1386 {
                          selector: w1386 -> [w1449 _]
                          tunnel: ["0" "4"] -> w1385
                          tunnel: [w1449 errorcluster {"status"=FALSE, "code"=0, "source"=""} ("error IO")] -> w1383
                          frame No Error {
                          }
                          frame Error {
                          }
                        }
                        n323 = flat-sequence {
                          tunnel: w1383 -> [w1522]
                          tunnel: [w1522] -> w1424
                          tunnel: [w1521] -> w1423
                          tunnel: w1414 -> [w1520]
                          tunnel: w1413 -> [w1519]
                          tunnel: [w1518] -> w1412
                          tunnel: [w1517] -> w1411
                          tunnel: w1403 -> [w1516]
                          tunnel: w1402 -> [w1515]
                          tunnel: w1401 -> [w1514]
                          tunnel: w1400 -> [w1513]
                          tunnel: w1399 -> [w1512]
                          tunnel: w1398 -> [w1511]
                          tunnel: w1385 -> [w1510]
                          tunnel: [w1510] -> w1384
                          frame #0 {
                            n324 = Build Array (concatenate)(w1520, w1516, w1515, w1514) -> (w1517:string[][])
                            n325 = Build Array (concatenate)(w1519, w1513, w1512, w1511) -> (w1518:string[][])
                            n326 = Select(t=Test_Sequences."Save Data" ("Test Sequences"), s=w1522, f=Test_Sequences."Close State VCmiin" ("Test Sequences")) -> (s? t:f=w1521:T8)
                          }
                        }
                      }
                      frame "Close State VCmiin" {
                        w1537 = FALSE ("true")
                        n327 = call "WS1021 CS Beam VCmin.vi"("Reg"=string[] ["43", "42", "43", "43", "43", "43", "43", "43", "42", "42", "42", "42", "42", "42"], "Error In"=w1553, "Cmd Bit"=string[] ["40", "40", "20", "01", "02", "04", "08", "10", "01", "02", "04", "08", "10", "20"], "Driver Name"=string[] ["FB1", "FB2", "FB3", "TB1", "TB2", "TB3", "TB4", "TB5", "TB6", "TB7", "TB8", "TB9", "TB10", "TB11"]) -> ("Error Out"=w1552:errorcluster, "Beam Cmd"=w1550:string[], "CS_Driver Name"=w1551:string[])  [unwired: 5 in]
                        n328 = case shown="False" w1536 {
                          tunnel: w1552 -> [w1634 w1665]
                          tunnel: w1566 -> [w1635 w1675]
                          tunnel: w1565 -> [w1628 w1666]
                          tunnel: [w1633 w1674] -> w1546
                          tunnel: [w1635 w1673] -> w1563
                          tunnel: w1530 -> [_ w1672]
                          tunnel: [w1630 w1670] -> w1548
                          tunnel: [w1629 w1669] -> w1547
                          tunnel: w1551 -> [w1632 w1668]
                          tunnel: w1550 -> [_ w1667]
                          tunnel: [w1628 w1666] -> w1540
                          tunnel: w1534 -> [_ w1663]
                          tunnel: w1533 -> [_ w1662]
                          tunnel: w1526 -> [_ w1661]
                          tunnel: w1525 -> [_ w1660]
                          frame False {
                            w1631 = string[][] []
                            n329 = for {
                              shift-right: [w1640] -> w1633
                              shift-left: w1634 -> [w1649]
                              tunnel: w1628 -> [w1651] mode=indexing
                              tunnel: w1632 -> [w1646]
                              shift-right: [w1645] -> w1630
                              shift-left: w1631 -> [w1644]
                              shift-right: [w1643] -> w1629
                              shift-left: w1631 -> [w1642]
                              n330 = Number To Fractional String(number=w1651, precision (6)=i16 2) -> (F-format string=w1648:string)  [unwired: 2 in]
                              n331 = for {
                                N: 32 -> [_]
                                shift-right: [w1659] -> w1641
                                shift-left: w1649 -> [w1659]
                                tunnel: w1648 -> [w1658]
                                tunnel: [w1658] -> w1639 mode=indexing
                              }
                              n332 = for {
                                tunnel: w1646 -> [_] mode=indexing
                                shift-right: [w1653] -> w1640
                                shift-left: w1641 -> [w1654]
                                tunnel: [w1652] -> w1638 mode=indexing
                                n333 = for {
                                N: 32 -> [_]
                                tunnel: [""] -> w1652 mode=indexing
                                shift-right: [w1656] -> w1653
                                shift-left: w1654 -> [w1656]
                                }
                              }
                              n334 = Build Array (concatenate)(w1639, w1638) -> (w1636:string[][])
                              n335 = Build Array (concatenate)(w1639, w1638) -> (w1637:string[][])
                              n336 = Build Array (concatenate)(w1644, w1636) -> (w1645:string[][])
                              n337 = Build Array (concatenate)(w1642, w1637) -> (w1643:string[][])
                            }
                          }
                          frame True {
                            w1671 = string[][] []
                            n338 = call "WS1021 CP Setting.vi"("Manual Setting"=w1662, "FPGA"=w1663, "Error In"=w1665) -> ("Error Out"=w1664:errorcluster)  [unwired: 7 in, 1 out]
                            n339 = for {
                              tunnel: w1666 -> [w1712] mode=indexing
                              shift-right: [w1689] -> w1674
                              shift-left: w1664 -> [w1713]
                              tunnel: w1675 -> [w1710]
                              tunnel: w1668 -> [w1699]
                              tunnel: w1667 -> [w1697]
                              tunnel: [w1696] -> w1673
                              shift-right: [w1694] -> w1670
                              shift-left: w1671 -> [w1695]
                              tunnel: w1672 -> [w1693]
                              shift-right: [w1691] -> w1669
                              shift-left: w1671 -> [w1692]
                              tunnel: w1661 -> [w1681]
                              tunnel: w1660 -> [w1679]
                              i -> [w1690]
                              n340 = call "Ke2400 Configure Output.vi"("error in (no error)"=w1713, "Compliance  Level (0.1)"=0.1, "Output Level (0)"=w1712, "VISA resource name"=w1710) -> ("error out"=w1709:errorcluster, "VISA resource name out"=w1708:refnum<visa-resource-name>)  [unwired: 6 in]
                              n341 = Number To Fractional String(number=w1712, precision (6)=i16 2) -> (F-format string=w1701:string)  [unwired: 2 in]
                              n342 = call "Ke2400 Enable.vi"("error in (no error)"=w1709, "ON/OFF"=TRUE, "VISA In"=w1708) -> ("error out"=w1706:errorcluster, "VISA Out"=w1696:refnum<visa-resource-name>)  [unwired: 7 in]
                              n343 = call "Time Delay.vi"("Error In"=w1706, "Delay(ms)"=u32 100) -> ("Error Out"=w1704:errorcluster)  [unwired: 9 in]
                              n344 = for {
                                N: 32 -> [_]
                                shift-right: [w1754] -> w1700
                                shift-left: w1704 -> [w1754]
                                tunnel: w1701 -> [w1753]
                                tunnel: [w1753] -> w1686 mode=indexing
                              }
                              n345 = Concatenate Strings("Testing CS " ("string"), w1701) -> (w1698:string)
                              n346 = for {
                                tunnel: w1699 -> [w1749] mode=indexing
                                tunnel: w1698 -> [w1752]
                                shift-right: [w1741] -> w1680
                                shift-left: w1700 -> [w1747]
                                tunnel: w1697 -> [w1746] mode=indexing
                                tunnel: w1693 -> [w1744]
                                tunnel: [w1737] -> w1687 mode=indexing
                                tunnel: [w1736] -> w1688 mode=indexing
                                n347 = call <vilib>:"Space Constant.vi"() -> ("String"=w1750:string)
                                n348 = call "WSVCAP SHL Host TL RFFE Write - Multiple DUTs - Common Data.vi"("Data Out"=w1746, "error in"=w1747, "FPGA"=w1744, "Log (T)"=FALSE) -> ("error out"=w1745:errorcluster)  [unwired: 11 in]
                                n349 = Concatenate Strings(w1752, w1750, w1749) -> (w1751:string)
                                n350 = call "WS1021 ADI Read 64 DUT.vi"("FPGA"=w1744, "Error In"=w1745) -> ("Error Out"=w1742:errorcluster, "AD7747 Values"=w1740:string[][])  [unwired: 8 in]
                                n351 = local write "Status"(w1751) -> ()
                                n352 = Index Array(array=w1740, index (col)=2 ("disabled index (col)")) -> (element=w1736:string[])  [unwired: 1 in]
                                n353 = Index Array(array=w1740, index (col)=5 ("disabled index (col)")) -> (element=w1737:string[])  [unwired: 1 in]
                                n354 = call "Time Delay.vi"("Error In"=w1742, "Delay(ms)"=u32 10) -> ("Error Out"=w1741:errorcluster)  [unwired: 9 in]
                              }
                              n355 = case shown="False" w1681 {
                                tunnel: w1687 -> [_ w1726]
                                tunnel: w1686 -> [_ w1725]
                                tunnel: [string[][] [] w1724] -> w1683
                                tunnel: w1680 -> [w1721 w1723]
                                tunnel: [w1721 w1723] -> w1676
                                frame False {
                                }
                                frame True {
                                n356 = Build Array (concatenate)(w1725, w1726) -> (w1724:string[][])
                                }
                              }
                              n357 = case shown="False" w1679 {
                                tunnel: w1688 -> [_ w1720]
                                tunnel: w1686 -> [_ w1719]
                                tunnel: [string[][] [] w1718] -> w1682
                                tunnel: w1680 -> [w1716 w1717]
                                tunnel: [w1716 w1717] -> w1678
                                frame False {
                                }
                                frame True {
                                n358 = Build Array (concatenate)(w1719, w1720) -> (w1718:string[][])
                                }
                              }
                              n359 = Transpose 2D Array(2D array=w1683) -> (transposed array=w1685:string[][])
                              n360 = Transpose 2D Array(2D array=w1682) -> (transposed array=w1684:string[][])
                              n361 = Merge Errors(w1676, w1678) -> (w1677:errorcluster)
                              n362 = case shown="1" w1690 {
                                tunnel: w1677 -> [w1729 w1732 w1735]
                                tunnel: [w1729 w1732 w1735] -> w1689
                                tunnel: w1685 -> [w1728 w1730 w1734]
                                tunnel: w1684 -> [w1727 w1731 w1733]
                                frame 0, Default {
                                "Brd B_CS_V1 (fF)" <- w1728
                                "Brd A_CS_V1 (fF)" <- w1727
                                }
                                frame 1 {
                                "Brd B_CS_V2 (fF)" <- w1730
                                "Brd A_CS_V2 (fF)" <- w1731
                                }
                                frame 2 {
                                "Brd B_CS_V3 (fF)" <- w1734
                                "Brd A_CS_V3 (fF)" <- w1733
                                }
                              }
                              n363 = Build Array (concatenate)(w1695, w1683) -> (w1694:string[][])
                              n364 = Build Array (concatenate)(w1692, w1682) -> (w1691:string[][])
                            }
                          }
                        }
                        n365 = Index Array(array=w1540, index=2) -> (element=w1535:dbl)
                        n366 = case shown="False" w1536 {
                          tunnel: w1546 -> [w1574 w1597]
                          tunnel: [w1573 w1596] -> w1545
                          tunnel: [w1575 w1595] -> w1532
                          tunnel: [w1576 w1594] -> w1539
                          tunnel: w1535 -> [_ w1592]
                          tunnel: [w1576 w1593] -> w1538
                          tunnel: w1535 -> [_ w1591]
                          tunnel: w1526 -> [_ w1590]
                          tunnel: w1525 -> [_ w1589]
                          frame False {
                            n367 = for {
                              N: 14 -> [_]
                              tunnel: [w1583] -> w1576 mode=indexing
                              shift-right: [w1581] -> w1575
                              shift-left: w1574 -> [w1582]
                              shift-right: [w1579] -> w1573
                              shift-left: w1574 -> [w1580]
                              n368 = for {
                                N: 31 -> [_]
                                tunnel: ["na"] -> w1585 mode=indexing
                                shift-right: [w1587] -> w1581
                                shift-left: w1582 -> [w1587]
                                shift-right: [w1586] -> w1579
                                shift-left: w1580 -> [w1586]
                              }
                              n369 = Build Array (concatenate)("na", w1585) -> (w1583:string[])
                            }
                          }
                          frame True {
                            n370 = case shown="False" w1590 {
                              tunnel: w1597 -> [w1608 w1615]
                              tunnel: [w1608 w1614] -> w1596
                              tunnel: [string[][] [] ("VCmin") w1610] -> w1594
                              tunnel: w1592 -> [_ w1609]
                              frame False {
                              }
                              frame True {
                                n371 = local read "Brd B_CS_V1 (fF)"() -> (w1613:string[][])
                                n372 = local read "Brd B_CS_V2 (fF)"() -> (w1612:string[][])
                                n373 = local read "Brd B_CS_V3 (fF)"() -> (w1611:string[][])
                                n374 = call "WS102x_Multi DUT_Calculate VCMIN.vi"("Pos_Voltage(V)"=w1609, "error in (no error)"=w1615, "V3_VCmin"=w1611, "V2_VCmin"=w1612, "V1_VCmin"=w1613) -> ("error out"=w1614:errorcluster, "VCmin"=w1610:string[][])  [unwired: 5 in]
                              }
                            }
                            n375 = case shown="True" w1589 {
                              tunnel: w1597 -> [w1599 w1606]
                              tunnel: [w1599 w1605] -> w1595
                              tunnel: [string[][] [] ("VCmin") w1601] -> w1593
                              tunnel: w1591 -> [_ w1600]
                              frame False {
                              }
                              frame True {
                                n376 = local read "Brd A_CS_V1 (fF)"() -> (w1604:string[][])
                                n377 = local read "Brd A_CS_V2 (fF)"() -> (w1603:string[][])
                                n378 = local read "Brd A_CS_V3 (fF)"() -> (w1602:string[][])
                                n379 = call "WS102x_Multi DUT_Calculate VCMIN.vi"("Pos_Voltage(V)"=w1600, "error in (no error)"=w1606, "V3_VCmin"=w1602, "V2_VCmin"=w1603, "V1_VCmin"=w1604) -> ("error out"=w1605:errorcluster, "VCmin"=w1601:string[][])  [unwired: 5 in]
                              }
                            }
                          }
                        }
                        n380 = call "WSVCAP SHL Host TL RFFE Write - Multiple DUTs - Common Data.vi"("Data Out"="0701020000", "error in"=w1532, "FPGA"=w1530, "Log (T)"=FALSE) -> ("error out"=w1531:errorcluster)  [unwired: 11 in]
                        n381 = case shown="1, Default" w1549 {
                          tunnel: w1531 -> [w1616 w1622]
                          tunnel: [w1616 w1622] -> w1543
                          tunnel: w1539 -> [w1621 w1627]
                          tunnel: w1538 -> [w1619 w1625]
                          tunnel: w1545 -> [w1617 w1623]
                          tunnel: [w1617 w1623] -> w1542
                          frame 0 {
                            n382 = Transpose 2D Array(2D array=w1621) -> (transposed array=→"Brd B_CS VCmin_T0":string[][])
                            n383 = Transpose 2D Array(2D array=w1619) -> (transposed array=→"Brd A_CS VCmin_T0":string[][])
                          }
                          frame 1, Default {
                            n384 = Transpose 2D Array(2D array=w1627) -> (transposed array=→"Brd B_CS VCmin":string[][])
                            n385 = Transpose 2D Array(2D array=w1625) -> (transposed array=→"Brd A_CS VCmin":string[][])
                          }
                        }
                        n386 = Merge Errors(w1542, w1543) -> (w1544:errorcluster)
                        n387 = call "Ke2400 Configure Output.vi"("error in (no error)"=w1544, "Output Level (0)"=0.0, "VISA resource name"=w1563) -> ("error out"=w1564:errorcluster, "VISA resource name out"=w1562:refnum<visa-resource-name>)  [unwired: 7 in]
                        n388 = flat-sequence {
                          tunnel: w1564 -> [w1757]
                          tunnel: [w1756] -> w1571
                          tunnel: [Test_Sequences."Save Data" ("Test Sequences")] -> w1572
                          tunnel: w1560 -> [w1766]
                          tunnel: [w1765] -> w1559
                          tunnel: w1558 -> [w1764]
                          tunnel: [w1763] -> w1557
                          tunnel: w1548 -> [w1762]
                          tunnel: w1547 -> [w1761]
                          tunnel: w1539 -> [w1760]
                          tunnel: w1538 -> [w1759]
                          tunnel: [w1755] -> w1527
                          frame #0 {
                            n389 = case shown="Error" w1757 {
                              selector: w1757 -> [w1768 _]
                              tunnel: [w1768 errorcluster {"status"=FALSE, "code"=0, "source"=""} ("error IO")] -> w1756
                              tunnel: ["0" "4"] -> w1755
                              frame No Error {
                              }
                              frame Error {
                              }
                            }
                            n390 = Build Array (concatenate)(w1764, w1761, w1759) -> (w1763:string[][])
                            n391 = Build Array (concatenate)(w1766, w1762, w1760) -> (w1765:string[][])
                          }
                        }
                      }
                      frame "Save Data" {
                        w1786 = FALSE ("true")
                        n392 = for {
                          N: 32 -> [_]
                          shift-right: [w1819] -> w1802
                          shift-left: w1803 -> [w1819]
                          tunnel: w1800 -> [w1818]
                          tunnel: [w1818] -> w1776 mode=indexing
                          tunnel: w1799 -> [w1817]
                          tunnel: [w1817] -> w1798 mode=indexing
                          tunnel: w1797 -> [w1816]
                          tunnel: [w1816] -> w1796 mode=indexing
                        }
                        n393 = call "WS1021 Multi DUT Generate Header Ver1.0.vi"("Reg 3"=w1791, "VPI Name"=w1789, "Reg 2"=w1790, "Error In"=w1802) -> ("Header"=w1804:string[], "Error Out"=w1808:errorcluster)  [unwired: 10 in]
                        n394 = Build Array (concatenate)(w1777, w1776, w1798) -> (w1793:string[][])
                        n395 = case shown="False" w1774 {
                          tunnel: w1795 -> [_ w1865]
                          tunnel: w1808 -> [w1861 w1866]
                          tunnel: [w1861 w1867] -> w1780
                          tunnel: w1804 -> [_ w1864]
                          tunnel: w1787 -> [_ w1863]
                          tunnel: w1793 -> [_ w1862]
                          tunnel: [string[][] [] w1862] -> w1772
                          frame False {
                          }
                          frame True {
                            # "Save Data Brd B"
                            n396 = call "WS1021_32DUT_Save Data_Ver1.0.vi"("Header"=w1864, "File Name"=w1863, "error in (no error)"=w1866, "base path"=w1865, "Data In"=w1862) -> ("error out"=w1867:errorcluster)  [unwired: 13 in, 1 out]
                          }
                        }
                        "Data Board B" <- w1772
                        n397 = Build Array (concatenate)(w1778, w1776, w1796) -> (w1792:string[][])
                        n398 = case shown="False" w1775 {
                          tunnel: w1794 -> [_ w1857]
                          tunnel: w1808 -> [w1853 w1858]
                          tunnel: [w1853 w1859] -> w1783
                          tunnel: w1804 -> [_ w1856]
                          tunnel: w1788 -> [_ w1855]
                          tunnel: w1792 -> [_ w1854]
                          tunnel: [string[][] [] w1854] -> w1771
                          frame False {
                          }
                          frame True {
                            # "Save Data Brd A"
                            n399 = call "WS1021_32DUT_Save Data_Ver1.0.vi"("Header"=w1856, "File Name"=w1855, "error in (no error)"=w1858, "base path"=w1857, "Data In"=w1854) -> ("error out"=w1859:errorcluster)  [unwired: 13 in, 1 out]
                          }
                        }
                        "Data Board A" <- w1771
                        n400 = local write "Status"("Save Data and Plot" ("Status")) -> ()
                        n401 = call "Time Delay.vi"("Error In"=w1783, "Delay(ms)"=u32 250) -> ("Error Out"=w1784:errorcluster)  [unwired: 9 in]
                        n402 = call "Time Delay.vi"("Error In"=w1780, "Delay(ms)"=u32 250) -> ("Error Out"=w1781:errorcluster)  [unwired: 9 in]
                        n403 = flat-sequence {
                          tunnel: w1784 -> [w1831]
                          tunnel: w1781 -> [w1833]
                          tunnel: [w1832] -> w1807
                          tunnel: [w1830] -> w1806
                          tunnel: w1795 -> [w1828]
                          tunnel: w1794 -> [w1826]
                          tunnel: w1788 -> [w1823]
                          tunnel: w1787 -> [w1822]
                          tunnel: w1775 -> [w1821]
                          tunnel: w1774 -> [w1820]
                          frame #0 {
                            # "Plots"
                            n404 = case shown="False" w1821 {
                              tunnel: w1831 -> [w1835 w1842]
                              tunnel: [w1835 w1841] -> w1830
                              tunnel: "Col CMin" -> [_ w1840]
                              tunnel: "Plot" -> [_ w1839]
                              tunnel: w1826 -> [_ w1838]
                              tunnel: [dbl[][] [] ("Delta COFF Plot (fF)") w1837] -> w1824
                              tunnel: w1823 -> [_ w1836]
                              frame False {
                              }
                              frame True {
                                n405 = call "WS1021 Multi DUT COFF Plots.vi"("Col CMin"=w1840, "File Name"=w1836, "Plot"=w1839, "file path (dialog if empty)"=w1838, "Error In"=w1842) -> ("Delta COFF Plot (fF)"=w1837:dbl[][], "Error Out"=w1841:errorcluster)  [unwired: 9 in]
                              }
                            }
                            n406 = case shown="False" w1820 {
                              tunnel: w1833 -> [w1844 w1851]
                              tunnel: [w1844 w1850] -> w1832
                              tunnel: "Col CMin" -> [_ w1849]
                              tunnel: w1828 -> [_ w1848]
                              tunnel: "Plot" -> [_ w1847]
                              tunnel: [dbl[][] [] ("Delta COFF Plot (fF)") w1846] -> w1825
                              tunnel: w1822 -> [_ w1845]
                              frame False {
                              }
                              frame True {
                                n407 = call "WS1021 Multi DUT COFF Plots.vi"("Col CMin"=w1849, "File Name"=w1845, "Plot"=w1847, "file path (dialog if empty)"=w1848, "Error In"=w1851) -> ("Delta COFF Plot (fF)"=w1846:dbl[][], "Error Out"=w1850:errorcluster)  [unwired: 9 in]
                              }
                            }
                            n408 = local write "Board B"(w1825) -> ()
                            n409 = local write "Board A"(w1824) -> ()
                          }
                        }
                        n410 = Merge Errors(w1807, w1806) -> (w1805:errorcluster)
                        n411 = flat-sequence {
                          tunnel: w1805 -> [w1874]
                          tunnel: [w1874] -> w1815
                          tunnel: [Test_Sequences."Exit" ("Test Sequences")] -> w1814
                          tunnel: [""] -> w1773
                          frame #0 {
                            n412 = Get Date/Time In Seconds() -> (seconds since 1Jan1904=w1873:timestamp)
                            n413 = Get Date/Time String(seconds (now)=w1873, want seconds? (F)=TRUE) -> (date string=→"Last Run Date":string, time string=→"Last Run Time":string)  [unwired: 1 in]
                          }
                        }
                      }
                      frame "Exit", Default {
                        n414 = flat-sequence {
                          tunnel: w1904 -> [w1924]
                          tunnel: "Set TTF" -> [w1926]
                          tunnel: [w1925] -> w1902
                          tunnel: [w1924] -> w1901
                          tunnel: [w1923] -> w1890
                          tunnel: w1902 -> [w1937]
                          tunnel: w1901 -> [w1936]
                          tunnel: [w1935] -> w1887
                          tunnel: [w1934] -> w1900
                          tunnel: w1896 -> [w1933]
                          tunnel: [w1932] -> w1893
                          tunnel: w1895 -> [w1931]
                          tunnel: [w1930] -> w1894
                          tunnel: w1890 -> [w1929]
                          tunnel: [w1929] -> w1889
                          tunnel: [w1928] -> w1883
                          frame #0 {
                            n415 = local read "TTF Completed"() -> (w1923:u64)
                            n416 = Greater Or Equal?(x=w1923, y=w1926) -> (x >= y?=w1925:bool)
                          }
                          frame #1 {
                            n417 = case shown="True" w1937 {
                              tunnel: w1936 -> [w1940 w1949]
                              tunnel: [FALSE ("true") w1947] -> w1935
                              tunnel: [w1940 w1946] -> w1934
                              tunnel: w1933 -> [w1939 w1945]
                              tunnel: [w1939 w1944] -> w1932
                              tunnel: w1931 -> [w1938 w1943]
                              tunnel: [w1938 w1942] -> w1930
                              frame False {
                              }
                              frame True {
                                n418 = flat-sequence {
                                tunnel: w1949 -> [w1959]
                                tunnel: [w1955] -> w1948
                                tunnel: w1945 -> [w1954]
                                tunnel: [w1953] -> w1944
                                tunnel: w1943 -> [w1952]
                                tunnel: [w1951] -> w1942
                                tunnel: w1948 -> [w1965]
                                tunnel: [w1966] -> w1947
                                tunnel: [w1965] -> w1946
                                frame #0 {
                                w1950 = u16 0 items=["Voltage", "Current"] ("Source Mode  (0: Voltage)")
                                w1962 = 0.0 ("Voltage 1")
                                n419 = call "E3631A_Voltage Controller updated.vi"("VISA resource name"=w1952, "I_VDD(A)"=w1962, "Channel Controller"=T13."Voltage 1", "Voltage 1"=w1962, "Voltage 2"=3.3, "error in (no error)"=w1959, "I_3.3V (A)"=0.5) -> ("VISA resource name out"=w1951:refnum<visa-resource-name>, "error out"=w1957:errorcluster)  [unwired: 7 in]
                                n420 = call "Ke2400 Configure Output.vi"("Source Mode  (0: Voltage)"=w1950, "error in (no error)"=w1959, "Output Level (0)"=0.0, "VISA resource name"=w1954) -> ("error out"=w1956:errorcluster, "VISA resource name out"=w1953:refnum<visa-resource-name>)  [unwired: 6 in]
                                n421 = Merge Errors(w1956, w1957) -> (w1955:errorcluster)
                                }
                                frame #1 {
                                w1964 = "Completed!" ("message")
                                n422 = local write "Status"(w1964) -> ()
                                n423 = One Button Dialog(message=w1964) -> (true=w1966:bool)  [unwired: 1 in]
                                }
                                }
                              }
                            }
                            n424 = Number To Fractional String(number=w1929, precision (6)=i16 0) -> (F-format string=w1928:string)  [unwired: 2 in]
                          }
                        }
                        n425 = case shown="True" w1884 {
                          tunnel: w1900 -> [w1914 w1922]
                          tunnel: w1879 -> [_ w1921]
                          tunnel: w1899 -> [_ w1920]
                          tunnel: w1898 -> [_ w1919]
                          tunnel: w1897 -> [_ w1918]
                          tunnel: w1883 -> [_ w1917]
                          tunnel: w1876 -> [_ w1916]
                          tunnel: [w1914 w1915] -> w1882
                          frame False {
                          }
                          frame True {
                            n426 = call "Save Errors Status.vi"("Lot"=w1920, "Stress"=w1917, "Wafer"=w1919, "error in (no error)"=w1922, "File Name"=w1918, "Error Status"=w1916, "base path"=w1921) -> ("error out"=w1915:errorcluster)  [unwired: 4 in]
                          }
                        }
                        n427 = case shown="True" w1880 {
                          tunnel: w1883 -> [_ w1913]
                          tunnel: w1882 -> [w1905 w1912]
                          tunnel: [w1905 w1911] -> w1881
                          tunnel: w1879 -> [_ w1910]
                          tunnel: w1878 -> [_ w1909]
                          tunnel: w1877 -> [_ w1908]
                          tunnel: w1876 -> [_ w1907]
                          tunnel: w1875 -> [_ w1906]
                          frame False {
                          }
                          frame True {
                            n428 = call "Save Errors Status.vi"("Lot"=w1909, "Stress"=w1913, "Wafer"=w1908, "error in (no error)"=w1912, "File Name"=w1906, "Error Status"=w1907, "base path"=w1910) -> ("error out"=w1911:errorcluster)  [unwired: 4 in]
                          }
                        }
                      }
                    }
                    "Test Sequences" <- w306
                    n429 = local write "Data Board A"(w247) -> ()
                    n430 = Concatenate Strings(w242, w244) -> (w243:string)
                    n431 = local write "Data Board B"(w248) -> ()
                    n432 = local write "Error Status"(w243) -> ()
                    n433 = Or(x=w286, y=w287) -> (x .or. y?=w288:bool)
                    n434 = call "Time Delay.vi"("Error In"=w286, "Delay(ms)"=u32 10) -> ("Error Out"=w298:errorcluster)  [unwired: 9 in]
                  }
                  n435 = call "Time Delay.vi"("Error In"=w168, "Delay(ms)"=u32 100) -> ("Error Out"=w171:errorcluster)  [unwired: 9 in]
                  n436 = Compound Arithmetic op=OR(w168, w167, w166) -> (w169:bool)
                }
                "Status" <- "Idle...." ("Status")
              }
              frame True {
              }
            }
            n437 = local write "Abort Stress"(FALSE ("Abort Stress")) -> ()
            n438 = Or(x=w92, y=w91) -> (x .or. y?=w93:bool)
          }
        }
        frame Error {
          n439 = flat-sequence {
            tunnel: w2131 -> [w2133]
            tunnel: [w2133] -> w2130
            tunnel: [w2132] -> _
            frame #0 {
              n440 = One Button Dialog(message="Communication Errors?") -> (true=w2132:bool)  [unwired: 1 in]
            }
          }
        }
      }
    }
    frame #2 {
      n441 = call "TLTSP_Close.vi"("error in (no error)"=w2137, "VISA In"=w2154) -> ("error out"=w2140:errorcluster, "VISA Out"=w2144:refnum<visa-resource-name>)  [unwired: 8 in]
      n442 = call "WSVCAP SHL Host TL Close.vi"("error in"=w2137, "FPGA"=w2136) -> ("error out"=w2135:errorcluster)  [unwired: 13 in]
      n443 = call "Ke2400 Enable.vi"("error in (no error)"=w2137, "ON/OFF"=FALSE, "VISA In"=w2149) -> ("error out"=w2142:errorcluster, "VISA Out"=w2147:refnum<visa-resource-name>)  [unwired: 7 in]
      n444 = call "E3631A_Voltage Controller updated.vi"("VISA resource name"=w2153, "I_VDD(A)"=0.5, "Channel Controller"=T13."Voltage 1", "Voltage 1"=0.0, "error in (no error)"=w2137) -> ("VISA resource name out"=w2145:refnum<visa-resource-name>, "error out"=w2141:errorcluster)  [unwired: 9 in]
      n445 = Build Array(w2147, w2146, w2145, w2144) -> (w2143:refnum<visa-resource-name>[])
      n446 = Merge Errors(w2142, w2141, w2140, w2135) -> (w2139:errorcluster)
      n447 = for {
        tunnel: w2143 -> [w2158] mode=indexing
        tunnel: w2139 -> [w2157]
        tunnel: [w2156] -> w2138
        n448 = VISA Close(VISA resource name=w2158, error in (no error)=w2157) -> (error out=w2156:errorcluster)
        n449 = Wait (ms)(milliseconds to wait=u32 10) -> ()  [unwired: 1 out]
      }
    }
  }
  "Error Out" <- w15
